vi "main.vi"() -> ()   [LabVIEW 2015, in "lv-example-postgres.lvlib"]
uses:
  lv-example-postgres.lvlib
  private/_controls/timezone.ctl
  <vilib>/addons/database/Connection.llb/Conn ObjectReference.ctl
  <vilib>/addons/database/Connection.llb/Conn Execute.vi
  <vilib>/addons/database/Recordset.llb/Rec Destroy - Connection.vi
  <vilib>/addons/database/Connection.llb/DB Tools Open Connec (String).vi
  <vilib>/addons/database/Command.llb/Cmd Execute.vi
  <vilib>/addons/database/Recordset.llb/Rec Fetch Recordset Data (CR).vi
  <vilib>/addons/database/Recordset.llb/Rec Destroy - Command.vi
  <vilib>/addons/database/Command.llb/Cmd Delete.vi
  <vilib>/addons/database/Recordset.llb/Rec Fetch Recordset Data (R).vi
  <vilib>/addons/database/NI_Database_API.lvlib
panel:
  in  "port":string="5432"
  in  "database":string="postgres"
  in  "display_timezone":i32(ring)=185 items=["Zulu (00:00:00)", "Libya (02:00:00)", "Antarctica/Mawson (05:00:00)", "Antarctica/McMurdo (13:00:00)", "Antarctica/South_Pole (13:00:00)", "Antarctica/Casey (11:00:00)", "Antarctica/Vostok (06:00:00)", "Antarctica/Troll (00:00:00)", "Antarctica/Syowa (03:00:00)", "Antarctica/Macquarie (11:00:00)", "Antarctica/Palmer (-03:00:00)", "Antarctica/DumontDUrville (10:00:00)", "Antarctica/Rothera (-03:00:00)", "Antarctica/Davis (07:00:00)", "NZ-CHAT (13:45:00)", "GMT+0 (00:00:00)", "Cuba (-05:00:00)", "MET (01:00:00)", "Hongkong (08:00:00)", "Poland (01:00:00)", "EST5EDT (-05:00:00)", "EET (02:00:00)", "posix/Zulu (00:00:00)", "posix/Libya (02:00:00)", "posix/Antarctica/Mawson (05:00:00)", "posix/Antarctica/McMurdo (13:00:00)", "posix/Antarctica/South_Pole (13:00:00)", "posix/Antarctica/Casey (11:00:00)", "posix/Antarctica/Vostok (06:00:00)", "posix/Antarctica/Troll (00:00:00)", "posix/Antarctica/Syowa (03:00:00)", "posix/Antarctica/Macquarie (11:00:00)", "posix/Antarctica/Palmer (-03:00:00)", "posix/Antarctica/DumontDUrville (10:00:00)", "posix/Antarctica/Rothera (-03:00:00)", "posix/Antarctica/Davis (07:00:00)", "posix/NZ-CHAT (13:45:00)", "posix/GMT+0 (00:00:00)", "posix/Cuba (-05:00:00)", "posix/MET (01:00:00)", "posix/Hongkong (08:00:00)", "posix/Poland (01:00:00)", "posix/EST5EDT (-05:00:00)", "posix/EET (02:00:00)", "posix/UTC (00:00:00)", "posix/HST (-10:00:00)", "posix/CST6CDT (-06:00:00)", "posix/PRC (08:00:00)", "posix/GB-Eire (00:00:00)", "posix/Australia/Queensland (10:00:00)", "posix/Australia/Currie (11:00:00)", "posix/Australia/Tasmania (11:00:00)", "posix/Australia/South (10:30:00)", "posix/Australia/Victoria (11:00:00)", "posix/Australia/Eucla (08:45:00)", "posix/Australia/Darwin (09:30:00)", "posix/Australia/Hobart (11:00:00)", "posix/Australia/NSW (11:00:00)", "posix/Australia/North (09:30:00)", "posix/Australia/Sydney (11:00:00)", "posix/Australia/Brisbane (10:00:00)", "posix/Australia/Lord_Howe (11:00:00)", "posix/Australia/Perth (08:00:00)", "posix/Australia/Melbourne (11:00:00)", "posix/Australia/LHI (11:00:00)", "posix/Australia/Yancowinna (10:30:00)", "posix/Australia/Lindeman (10:00:00)", "posix/Australia/ACT (11:00:00)", "posix/Australia/Broken_Hill (10:30:00)", "posix/Australia/West (08:00:00)", "posix/Australia/Adelaide (10:30:00)", "posix/Australia/Canberra (11:00:00)", "posix/Europe/Busingen (01:00:00)", "posix/Europe/Gibraltar (01:00:00)", "posix/Europe/San_Marino (01:00:00)", "posix/Europe/Madrid (01:00:00)", "posix/Europe/Helsinki (02:00:00)", "posix/Europe/Brussels (01:00:00)", "posix/Europe/Astrakhan (04:00:00)", "posix/Europe/Belfast (00:00:00)", "posix/Europe/Uzhgorod (02:00:00)", "posix/Europe/Riga (02:00:00)", "posix/Europe/Sarajevo (01:00:00)", "posix/Europe/Vienna (01:00:00)", "posix/Europe/London (00:00:00)", "posix/Europe/Lisbon (00:00:00)", "posix/Europe/Skopje (01:00:00)", "posix/Europe/Monaco (01:00:00)", "posix/Europe/Vaduz (01:00:00)", "posix/Europe/Amsterdam (01:00:00)", "posix/Europe/Kiev (02:00:00)", "posix/Europe/Vilnius (02:00:00)", "posix/Europe/Oslo (01:00:00)", "posix/Europe/Nicosia (02:00:00)", "posix/Europe/Minsk (03:00:00)", "posix/Europe/Budapest (01:00:00)", "posix/Europe/Samara (04:00:00)", "posix/Europe/Kirov (03:00:00)", "posix/Europe/Kaliningrad (02:00:00)", "posix/Europe/Ljubljana (01:00:00)", "posix/Europe/Simferopol (03:00:00)", "posix/Europe/Tiraspol (02:00:00)", "posix/Europe/Stockholm (01:00:00)", "posix/Europe/Isle_of_Man (00:00:00)", "posix/Europe/Guernsey (00:00:00)", "posix/Europe/Belgrade (01:00:00)", "posix/Europe/Zagreb (01:00:00)", "posix/Europe/Rome (01:00:00)", "posix/Europe/Berlin (01:00:00)", "posix/Europe/Ulyanovsk (04:00:00)", "posix/Europe/Mariehamn (02:00:00)", "posix/Europe/Bucharest (02:00:00)", "posix/Europe/Warsaw (01:00:00)", "posix/Europe/Vatican (01:00:00)", "posix/Europe/Dublin (00:00:00)", "posix/Europe/Istanbul (03:00:00)", "posix/Europe/Andorra (01:00:00)", "posix/Europe/Chisinau (02:00:00)", "posix/Europe/Jersey (00:00:00)", "posix/Europe/Zurich (01:00:00)", "posix/Europe/Athens (02:00:00)", "posix/Europe/Paris (01:00:00)", "posix/Europe/Saratov (04:00:00)", "posix/Europe/Prague (01:00:00)", "posix/Europe/Bratislava (01:00:00)", "posix/Europe/Malta (01:00:00)", "posix/Europe/Podgorica (01:00:00)", "posix/Europe/Copenhagen (01:00:00)", "posix/Europe/Moscow (03:00:00)", "posix/Europe/Luxembourg (01:00:00)", "posix/Europe/Zaporozhye (02:00:00)", "posix/Europe/Tirane (01:00:00)", "posix/Europe/Tallinn (02:00:00)", "posix/Europe/Sofia (02:00:00)", "posix/Europe/Volgograd (03:00:00)", "posix/EST (-05:00:00)", "posix/GMT-0 (00:00:00)", "posix/GMT (00:00:00)", "posix/Navajo (-07:00:00)", "posix/Eire (00:00:00)", "posix/Africa/Dar_es_Salaam (03:00:00)", "posix/Africa/Monrovia (00:00:00)", "posix/Africa/Bissau (00:00:00)", "posix/Africa/Juba (02:00:00)", "posix/Africa/Kinshasa (01:00:00)", "posix/Africa/Mogadishu (03:00:00)", "posix/Africa/Ceuta (01:00:00)", "posix/Africa/Asmara (03:00:00)", "posix/Africa/Asmera (03:00:00)", "posix/Africa/Timbuktu (00:00:00)", "posix/Africa/Tripoli (02:00:00)", "posix/Africa/Blantyre (02:00:00)", "posix/Africa/Banjul (00:00:00)", "posix/Africa/Khartoum (02:00:00)", "posix/Africa/Brazzaville (01:00:00)", "posix/Africa/Ouagadougou (00:00:00)", "posix/Africa/Luanda (01:00:00)", "posix/Africa/Conakry (00:00:00)", "posix/Africa/Tunis (01:00:00)", "posix/Africa/Freetown (00:00:00)", "posix/Africa/Maseru (02:00:00)", "posix/Africa/Addis_Ababa (03:00:00)", "posix/Africa/Abidjan (00:00:00)", "posix/Africa/Maputo (02:00:00)", "posix/Africa/Windhoek (02:00:00)", "posix/Africa/Djibouti (03:00:00)", "posix/Africa/Nouakchott (00:00:00)", "posix/Africa/Cairo (02:00:00)", "posix/Africa/Ndjamena (01:00:00)", "posix/Africa/Nairobi (03:00:00)", "posix/Africa/Harare (02:00:00)", "posix/Africa/Bangui (01:00:00)", "posix/Africa/Lome (00:00:00)", "posix/Africa/Lusaka (02:00:00)", "posix/Africa/Lubumbashi (02:00:00)", "posix/Africa/Douala (01:00:00)", "posix/Africa/Bujumbura (02:00:00)", "posix/Africa/Lagos (01:00:00)", "posix/Africa/Dakar (00:00:00)", "posix/Africa/Porto-Novo (01:00:00)", "posix/Africa/Mbabane (02:00:00)", "posix/Africa/Accra (00:00:00)", "posix/Africa/Kigali (02:00:00)", "posix/Africa/Casablanca (01:00:00)", "posix/Africa/Algiers (01:00:00)", "posix/Africa/Malabo (01:00:00)", "posix/Africa/Niamey (01:00:00)", "posix/Africa/Sao_Tome (00:00:00)", "posix/Africa/Libreville (01:00:00)", "posix/Africa/Bamako (00:00:00)", "posix/Africa/El_Aaiun (01:00:00)", "posix/Africa/Gaborone (02:00:00)", "posix/Africa/Johannesburg (02:00:00)", "posix/Africa/Kampala (03:00:00)", "posix/NZ (13:00:00)", "posix/MST (-07:00:00)", "posix/Arctic/Longyearbyen (01:00:00)", "posix/Turkey (03:00:00)", "posix/US/Indiana-Starke (-06:00:00)", "posix/US/Michigan (-05:00:00)", "posix/US/Hawaii (-10:00:00)", "posix/US/East-Indiana (-05:00:00)", "posix/US/Samoa (-11:00:00)", "posix/US/Alaska (-09:00:00)", "posix/US/Aleutian (-10:00:00)", "posix/US/Arizona (-07:00:00)", "posix/US/Mountain (-07:00:00)", "posix/US/Central (-06:00:00)", "posix/US/Eastern (-05:00:00)", "posix/US/Pacific (-08:00:00)", "posix/Canada/Yukon (-07:00:00)", "posix/Canada/Newfoundland (-02:30:00)", "posix/Canada/Atlantic (-04:00:00)", "posix/Canada/Mountain (-07:00:00)", "posix/Canada/Saskatchewan (-06:00:00)", "posix/Canada/Central (-06:00:00)", "posix/Canada/Eastern (-05:00:00)", "posix/Canada/Pacific (-08:00:00)", "posix/Iceland (00:00:00)", "posix/Israel (02:00:00)", "posix/GMT0 (00:00:00)", "posix/Brazil/East (-03:00:00)", "posix/Brazil/Acre (-05:00:00)", "posix/Brazil/DeNoronha (-02:00:00)", "posix/Brazil/West (-04:00:00)", "posix/Japan (09:00:00)", "posix/ROK (09:00:00)", "posix/Atlantic/Faeroe (00:00:00)", "posix/Atlantic/Jan_Mayen (01:00:00)", "posix/Atlantic/Faroe (00:00:00)", "posix/Atlantic/Madeira (00:00:00)", "posix/Atlantic/St_Helena (00:00:00)", "posix/Atlantic/Canary (00:00:00)", "posix/Atlantic/Reykjavik (00:00:00)", "posix/Atlantic/South_Georgia (-02:00:00)", "posix/Atlantic/Stanley (-03:00:00)", "posix/Atlantic/Cape_Verde (-01:00:00)", "posix/Atlantic/Azores (-01:00:00)", "posix/Atlantic/Bermuda (-04:00:00)", "posix/ROC (08:00:00)", "posix/MST7MDT (-07:00:00)", "posix/America/Eirunepe (-05:00:00)", "posix/America/Danmarkshavn (00:00:00)", "posix/America/Santo_Domingo (-04:00:00)", "posix/America/Chicago (-06:00:00)", "posix/America/Jujuy (-03:00:00)", "posix/America/Regina (-06:00:00)", "posix/America/Atikokan (-05:00:00)", "posix/America/Porto_Velho (-04:00:00)", "posix/America/Port_of_Spain (-04:00:00)", "posix/America/Kentucky/Monticello (-05:00:00)", "posix/America/Kentucky/Louisville (-05:00:00)", "posix/America/Anguilla (-04:00:00)", "posix/America/Tegucigalpa (-06:00:00)", "posix/America/Panama (-05:00:00)", "posix/America/Antigua (-04:00:00)", "posix/America/Cancun (-05:00:00)", "posix/America/Araguaina (-03:00:00)", "posix/America/Goose_Bay (-04:00:00)", "posix/America/Coral_Harbour (-05:00:00)", "posix/America/Nipigon (-05:00:00)", "posix/America/New_York (-05:00:00)", "posix/America/Merida (-06:00:00)", "posix/America/Martinique (-04:00:00)", "posix/America/Inuvik (-07:00:00)", "posix/America/Nassau (-05:00:00)", "posix/America/Cuiaba (-04:00:00)", "posix/America/Phoenix (-07:00:00)", "posix/America/Costa_Rica (-06:00:00)", "posix/America/Toronto (-05:00:00)", "posix/America/Guadeloupe (-04:00:00)", "posix/America/Argentina/Jujuy (-03:00:00)", "posix/America/Argentina/Ushuaia (-03:00:00)", "posix/America/Argentina/Rio_Gallegos (-03:00:00)", "posix/America/Argentina/San_Luis (-03:00:00)", "posix/America/Argentina/San_Juan (-03:00:00)", "posix/America/Argentina/Salta (-03:00:00)", "posix/America/Argentina/La_Rioja (-03:00:00)", "posix/America/Argentina/Catamarca (-03:00:00)", "posix/America/Argentina/ComodRivadavia (-03:00:00)", "posix/America/Argentina/Buenos_Aires (-03:00:00)", "posix/America/Argentina/Cordoba (-03:00:00)", "posix/America/Argentina/Tucuman (-03:00:00)", "posix/America/Argentina/Mendoza (-03:00:00)", "posix/America/Mazatlan (-07:00:00)", "posix/America/Paramaribo (-03:00:00)", "posix/America/Nuuk (-03:00:00)", "posix/America/Thule (-04:00:00)", "posix/America/Sao_Paulo (-03:00:00)", "posix/America/Managua (-06:00:00)", "posix/America/Moncton (-04:00:00)", "posix/America/Recife (-03:00:00)", "posix/America/Port-au-Prince (-05:00:00)", "posix/America/Marigot (-04:00:00)", "posix/America/Anchorage (-09:00:00)", "posix/America/Knox_IN (-06:00:00)", "posix/America/Cayenne (-03:00:00)", "posix/America/Mexico_City (-06:00:00)", "posix/America/Santa_Isabel (-08:00:00)", "posix/America/Glace_Bay (-04:00:00)", "posix/America/Chihuahua (-07:00:00)", "posix/America/Montreal (-05:00:00)", "posix/America/Guayaquil (-05:00:00)", "posix/America/Noronha (-02:00:00)", "posix/America/Dawson (-07:00:00)", "posix/America/Belem (-03:00:00)", "posix/America/Guyana (-04:00:00)", "posix/America/Guatemala (-06:00:00)", "posix/America/Boa_Vista (-04:00:00)", "posix/America/St_Vincent (-04:00:00)", "posix/America/Aruba (-04:00:00)", "posix/America/Rosario (-03:00:00)", "posix/America/Matamoros (-06:00:00)", "posix/America/Detroit (-05:00:00)", "posix/America/Lower_Princes (-04:00:00)", "posix/America/St_Barthelemy (-04:00:00)", "posix/America/St_Johns (-02:30:00)", "posix/America/Tortola (-04:00:00)", "posix/America/Rankin_Inlet (-06:00:00)", "posix/America/Blanc-Sablon (-04:00:00)", "posix/America/Punta_Arenas (-03:00:00)", "posix/America/Bahia (-03:00:00)", "posix/America/Godthab (-03:00:00)", "posix/America/Halifax (-04:00:00)", "posix/America/Virgin (-04:00:00)", "posix/America/Grand_Turk (-05:00:00)", "posix/America/Scoresbysund (-01:00:00)", "posix/America/Ojinaga (-07:00:00)", "posix/America/Nome (-09:00:00)", "posix/America/Havana (-05:00:00)", "posix/America/Thunder_Bay (-05:00:00)", "posix/America/Bogota (-05:00:00)", "posix/America/Belize (-06:00:00)", "posix/America/Tijuana (-08:00:00)", "posix/America/Sitka (-09:00:00)", "posix/America/Juneau (-09:00:00)", "posix/America/Shiprock (-07:00:00)", "posix/America/Porto_Acre (-05:00:00)", "posix/America/Monterrey (-06:00:00)", "posix/America/Winnipeg (-06:00:00)", "posix/America/Boise (-07:00:00)", "posix/America/Iqaluit (-05:00:00)", "posix/America/Puerto_Rico (-04:00:00)", "posix/America/Santarem (-03:00:00)", "posix/America/Curacao (-04:00:00)", "posix/America/North_Dakota/Center (-06:00:00)", "posix/America/North_Dakota/New_Salem (-06:00:00)", "posix/America/North_Dakota/Beulah (-06:00:00)", "posix/America/El_Salvador (-06:00:00)", "posix/America/Menominee (-06:00:00)", "posix/America/Montserrat (-04:00:00)", "posix/America/Indianapolis (-05:00:00)", "posix/America/Rainy_River (-06:00:00)", "posix/America/Dominica (-04:00:00)", "posix/America/Fortaleza (-03:00:00)", "posix/America/Cambridge_Bay (-07:00:00)", "posix/America/Fort_Nelson (-07:00:00)", "posix/America/St_Kitts (-04:00:00)", "posix/America/Yellowknife (-07:00:00)", "posix/America/Santiago (-03:00:00)", "posix/America/Maceio (-03:00:00)", "posix/America/Louisville (-05:00:00)", "posix/America/Catamarca (-03:00:00)", "posix/America/Bahia_Banderas (-06:00:00)", "posix/America/Campo_Grande (-04:00:00)", "posix/America/St_Lucia (-04:00:00)", "posix/America/Buenos_Aires (-03:00:00)", "posix/America/Asuncion (-03:00:00)", "posix/America/Hermosillo (-07:00:00)", "posix/America/Cordoba (-03:00:00)", "posix/America/Edmonton (-07:00:00)", "posix/America/Barbados (-04:00:00)", "posix/America/Lima (-05:00:00)", "posix/America/Dawson_Creek (-07:00:00)", "posix/America/Manaus (-04:00:00)", "posix/America/Yakutat (-09:00:00)", "posix/America/Pangnirtung (-05:00:00)", "posix/America/Caracas (-04:00:00)", "posix/America/Rio_Branco (-05:00:00)", "posix/America/Creston (-07:00:00)", "posix/America/Grenada (-04:00:00)", "posix/America/La_Paz (-04:00:00)", "posix/America/Adak (-10:00:00)", "posix/America/Los_Angeles (-08:00:00)", "posix/America/Fort_Wayne (-05:00:00)", "posix/America/Montevideo (-03:00:00)", "posix/America/Whitehorse (-07:00:00)", "posix/America/Jamaica (-05:00:00)", "posix/America/Mendoza (-03:00:00)", "posix/America/Kralendijk (-04:00:00)", "posix/America/St_Thomas (-04:00:00)", "posix/America/Vancouver (-08:00:00)", "posix/America/Ensenada (-08:00:00)", "posix/America/Metlakatla (-09:00:00)", "posix/America/Indiana/Marengo (-05:00:00)", "posix/America/Indiana/Knox (-06:00:00)", "posix/America/Indiana/Tell_City (-06:00:00)", "posix/America/Indiana/Vevay (-05:00:00)", "posix/America/Indiana/Winamac (-05:00:00)", "posix/America/Indiana/Indianapolis (-05:00:00)", "posix/America/Indiana/Vincennes (-05:00:00)", "posix/America/Indiana/Petersburg (-05:00:00)", "posix/America/Cayman (-05:00:00)", "posix/America/Miquelon (-03:00:00)", "posix/America/Swift_Current (-06:00:00)", "posix/America/Resolute (-06:00:00)", "posix/America/Atka (-10:00:00)", "posix/America/Denver (-07:00:00)", "posix/Universal (00:00:00)", "posix/Etc/Zulu (00:00:00)", "posix/Etc/GMT+0 (00:00:00)", "posix/Etc/GMT-12 (12:00:00)", "posix/Etc/GMT-13 (13:00:00)", "posix/Etc/GMT-6 (06:00:00)", "posix/Etc/UTC (00:00:00)", "posix/Etc/GMT-10 (10:00:00)", "posix/Etc/GMT-3 (03:00:00)", "posix/Etc/GMT-0 (00:00:00)", "posix/Etc/GMT-11 (11:00:00)", "posix/Etc/GMT-5 (05:00:00)", "posix/Etc/GMT (00:00:00)", "posix/Etc/GMT-4 (04:00:00)", "posix/Etc/GMT+3 (-03:00:00)", "posix/Etc/GMT+2 (-02:00:00)", "posix/Etc/GMT0 (00:00:00)", "posix/Etc/GMT-1 (01:00:00)", "posix/Etc/Universal (00:00:00)", "posix/Etc/GMT+7 (-07:00:00)", "posix/Etc/GMT-14 (14:00:00)", "posix/Etc/GMT+1 (-01:00:00)", "posix/Etc/Greenwich (00:00:00)", "posix/Etc/GMT+12 (-12:00:00)", "posix/Etc/GMT-2 (02:00:00)", "posix/Etc/GMT+8 (-08:00:00)", "posix/Etc/GMT+9 (-09:00:00)", "posix/Etc/GMT+11 (-11:00:00)", "posix/Etc/UCT (00:00:00)", "posix/Etc/GMT-8 (08:00:00)", "posix/Etc/GMT+6 (-06:00:00)", "posix/Etc/GMT+10 (-10:00:00)", "posix/Etc/GMT+5 (-05:00:00)", "posix/Etc/GMT-9 (09:00:00)", "posix/Etc/GMT+4 (-04:00:00)", "posix/Etc/GMT-7 (07:00:00)", "posix/Indian/Mayotte (03:00:00)", "posix/Indian/Chagos (06:00:00)", "posix/Indian/Christmas (07:00:00)", "posix/Indian/Cocos (06:30:00)", "posix/Indian/Reunion (04:00:00)", "posix/Indian/Mahe (04:00:00)", "posix/Indian/Maldives (05:00:00)", "posix/Indian/Comoro (03:00:00)", "posix/Indian/Kerguelen (05:00:00)", "posix/Indian/Antananarivo (03:00:00)", "posix/Indian/Mauritius (04:00:00)", "posix/Kwajalein (12:00:00)", "posix/Greenwich (00:00:00)", "posix/W-SU (03:00:00)", "posix/UCT (00:00:00)", "posix/Iran (03:30:00)", "posix/Egypt (02:00:00)", "posix/Chile/Continental (-03:00:00)", "posix/Chile/EasterIsland (-05:00:00)", "posix/Asia/Bangkok (07:00:00)", "posix/Asia/Srednekolymsk (11:00:00)", "posix/Asia/Phnom_Penh (07:00:00)", "posix/Asia/Gaza (02:00:00)", "posix/Asia/Qyzylorda (05:00:00)", "posix/Asia/Aden (03:00:00)", "posix/Asia/Chungking (08:00:00)", "posix/Asia/Ulaanbaatar (08:00:00)", "posix/Asia/Kuwait (03:00:00)", "posix/Asia/Dushanbe (05:00:00)", "posix/Asia/Shanghai (08:00:00)", "posix/Asia/Novokuznetsk (07:00:00)", "posix/Asia/Pontianak (07:00:00)", "posix/Asia/Bahrain (03:00:00)", "posix/Asia/Brunei (08:00:00)", "posix/Asia/Dhaka (06:00:00)", "posix/Asia/Bishkek (06:00:00)", "posix/Asia/Barnaul (07:00:00)", "posix/Asia/Ho_Chi_Minh (07:00:00)", "posix/Asia/Macau (08:00:00)", "posix/Asia/Pyongyang (09:00:00)", "posix/Asia/Ashkhabad (05:00:00)", "posix/Asia/Kuala_Lumpur (08:00:00)", "posix/Asia/Yangon (06:30:00)", "posix/Asia/Magadan (11:00:00)", "posix/Asia/Ashgabat (05:00:00)", "posix/Asia/Saigon (07:00:00)", "posix/Asia/Calcutta (05:30:00)", "posix/Asia/Tel_Aviv (02:00:00)", "posix/Asia/Karachi (05:00:00)", "posix/Asia/Atyrau (05:00:00)", "posix/Asia/Samarkand (05:00:00)", "posix/Asia/Taipei (08:00:00)", "posix/Asia/Aqtobe (05:00:00)", "posix/Asia/Riyadh (03:00:00)", "posix/Asia/Almaty (06:00:00)", "posix/Asia/Jakarta (07:00:00)", "posix/Asia/Manila (08:00:00)", "posix/Asia/Nicosia (02:00:00)", "posix/Asia/Novosibirsk (07:00:00)", "posix/Asia/Tokyo (09:00:00)", "posix/Asia/Thimphu (06:00:00)", "posix/Asia/Vientiane (07:00:00)", "posix/Asia/Ulan_Bator (08:00:00)", "posix/Asia/Anadyr (12:00:00)", "posix/Asia/Hovd (07:00:00)", "posix/Asia/Dacca (06:00:00)", "posix/Asia/Beirut (02:00:00)", "posix/Asia/Irkutsk (08:00:00)", "posix/Asia/Yakutsk (09:00:00)", "posix/Asia/Kabul (04:30:00)", "posix/Asia/Tehran (03:30:00)", "posix/Asia/Hong_Kong (08:00:00)", "posix/Asia/Macao (08:00:00)", "posix/Asia/Urumqi (06:00:00)", "posix/Asia/Muscat (04:00:00)", "posix/Asia/Thimbu (06:00:00)", "posix/Asia/Chita (09:00:00)", "posix/Asia/Tomsk (07:00:00)", "posix/Asia/Aqtau (05:00:00)", "posix/Asia/Krasnoyarsk (07:00:00)", "posix/Asia/Kashgar (06:00:00)", "posix/Asia/Kolkata (05:30:00)", "posix/Asia/Kathmandu (05:45:00)", "posix/Asia/Sakhalin (11:00:00)", "posix/Asia/Oral (05:00:00)", "posix/Asia/Tashkent (05:00:00)", "posix/Asia/Istanbul (03:00:00)", "posix/Asia/Dili (09:00:00)", "posix/Asia/Jayapura (09:00:00)", "posix/Asia/Qostanay (06:00:00)", "posix/Asia/Khandyga (09:00:00)", "posix/Asia/Vladivostok (10:00:00)", "posix/Asia/Seoul (09:00:00)", "posix/Asia/Harbin (08:00:00)", "posix/Asia/Amman (02:00:00)", "posix/Asia/Ust-Nera (10:00:00)", "posix/Asia/Qatar (03:00:00)", "posix/Asia/Kuching (08:00:00)", "posix/Asia/Omsk (06:00:00)", "posix/Asia/Baghdad (03:00:00)", "posix/Asia/Choibalsan (08:00:00)", "posix/Asia/Dubai (04:00:00)", "posix/Asia/Chongqing (08:00:00)", "posix/Asia/Makassar (08:00:00)", "posix/Asia/Rangoon (06:30:00)", "posix/Asia/Singapore (08:00:00)", "posix/Asia/Yerevan (04:00:00)", "posix/Asia/Damascus (02:00:00)", "posix/Asia/Tbilisi (04:00:00)", "posix/Asia/Katmandu (05:45:00)", "posix/Asia/Baku (04:00:00)", "posix/Asia/Yekaterinburg (05:00:00)", "posix/Asia/Hebron (02:00:00)", "posix/Asia/Famagusta (02:00:00)", "posix/Asia/Ujung_Pandang (08:00:00)", "posix/Asia/Colombo (05:30:00)", "posix/Asia/Kamchatka (12:00:00)", "posix/Asia/Jerusalem (02:00:00)", "posix/GB (00:00:00)", "posix/Singapore (08:00:00)", "posix/CET (01:00:00)", "posix/Jamaica (-05:00:00)", "posix/PST8PDT (-08:00:00)", "posix/Portugal (00:00:00)", "posix/Pacific/Efate (11:00:00)", "posix/Pacific/Yap (10:00:00)", "posix/Pacific/Wallis (12:00:00)", "posix/Pacific/Saipan (10:00:00)", "posix/Pacific/Tahiti (-10:00:00)", "posix/Pacific/Bougainville (11:00:00)", "posix/Pacific/Pago_Pago (-11:00:00)", "posix/Pacific/Niue (-11:00:00)", "posix/Pacific/Honolulu (-10:00:00)", "posix/Pacific/Samoa (-11:00:00)", "posix/Pacific/Enderbury (13:00:00)", "posix/Pacific/Pitcairn (-08:00:00)", "posix/Pacific/Johnston (-10:00:00)", "posix/Pacific/Funafuti (12:00:00)", "posix/Pacific/Norfolk (12:00:00)", "posix/Pacific/Tongatapu (13:00:00)", "posix/Pacific/Apia (13:00:00)", "posix/Pacific/Truk (10:00:00)", "posix/Pacific/Guam (10:00:00)", "posix/Pacific/Nauru (12:00:00)", "posix/Pacific/Palau (09:00:00)", "posix/Pacific/Chatham (13:45:00)", "posix/Pacific/Rarotonga (-10:00:00)", "posix/Pacific/Majuro (12:00:00)", "posix/Pacific/Wake (12:00:00)", "posix/Pacific/Gambier (-09:00:00)", "posix/Pacific/Auckland (13:00:00)", "posix/Pacific/Pohnpei (11:00:00)", "posix/Pacific/Midway (-11:00:00)", "posix/Pacific/Fiji (13:00:00)", "posix/Pacific/Marquesas (-08:30:00)", "posix/Pacific/Ponape (11:00:00)", "posix/Pacific/Port_Moresby (10:00:00)", "posix/Pacific/Noumea (11:00:00)", "posix/Pacific/Kwajalein (12:00:00)", "posix/Pacific/Tarawa (12:00:00)", "posix/Pacific/Easter (-05:00:00)", "posix/Pacific/Chuuk (10:00:00)", "posix/Pacific/Kiritimati (14:00:00)", "posix/Pacific/Guadalcanal (11:00:00)", "posix/Pacific/Galapagos (-06:00:00)", "posix/Pacific/Fakaofo (13:00:00)", "posix/Pacific/Kosrae (11:00:00)", "posix/Factory (00:00:00)", "posix/WET (00:00:00)", "posix/Mexico/BajaSur (-07:00:00)", "posix/Mexico/BajaNorte (-08:00:00)", "posix/Mexico/General (-06:00:00)", "UTC (00:00:00)", "HST (-10:00:00)", "CST6CDT (-06:00:00)", "PRC (08:00:00)", "GB-Eire (00:00:00)", "Australia/Queensland (10:00:00)", "Australia/Currie (11:00:00)", "Australia/Tasmania (11:00:00)", "Australia/South (10:30:00)", "Australia/Victoria (11:00:00)", "Australia/Eucla (08:45:00)", "Australia/Darwin (09:30:00)", "Australia/Hobart (11:00:00)", "Australia/NSW (11:00:00)", "Australia/North (09:30:00)", "Australia/Sydney (11:00:00)", "Australia/Brisbane (10:00:00)", "Australia/Lord_Howe (11:00:00)", "Australia/Perth (08:00:00)", "Australia/Melbourne (11:00:00)", "Australia/LHI (11:00:00)", "Australia/Yancowinna (10:30:00)", "Australia/Lindeman (10:00:00)", "Australia/ACT (11:00:00)", "Australia/Broken_Hill (10:30:00)", "Australia/West (08:00:00)", "Australia/Adelaide (10:30:00)", "Australia/Canberra (11:00:00)", "Europe/Busingen (01:00:00)", "Europe/Gibraltar (01:00:00)", "Europe/San_Marino (01:00:00)", "Europe/Madrid (01:00:00)", "Europe/Helsinki (02:00:00)", "Europe/Brussels (01:00:00)", "Europe/Astrakhan (04:00:00)", "Europe/Belfast (00:00:00)", "Europe/Uzhgorod (02:00:00)", "Europe/Riga (02:00:00)", "Europe/Sarajevo (01:00:00)", "Europe/Vienna (01:00:00)", "Europe/London (00:00:00)", "Europe/Lisbon (00:00:00)", "Europe/Skopje (01:00:00)", "Europe/Monaco (01:00:00)", "Europe/Vaduz (01:00:00)", "Europe/Amsterdam (01:00:00)", "Europe/Kiev (02:00:00)", "Europe/Vilnius (02:00:00)", "Europe/Oslo (01:00:00)", "Europe/Nicosia (02:00:00)", "Europe/Minsk (03:00:00)", "Europe/Budapest (01:00:00)", "Europe/Samara (04:00:00)", "Europe/Kirov (03:00:00)", "Europe/Kaliningrad (02:00:00)", "Europe/Ljubljana (01:00:00)", "Europe/Simferopol (03:00:00)", "Europe/Tiraspol (02:00:00)", "Europe/Stockholm (01:00:00)", "Europe/Isle_of_Man (00:00:00)", "Europe/Guernsey (00:00:00)", "Europe/Belgrade (01:00:00)", "Europe/Zagreb (01:00:00)", "Europe/Rome (01:00:00)", "Europe/Berlin (01:00:00)", "Europe/Ulyanovsk (04:00:00)", "Europe/Mariehamn (02:00:00)", "Europe/Bucharest (02:00:00)", "Europe/Warsaw (01:00:00)", "Europe/Vatican (01:00:00)", "Europe/Dublin (00:00:00)", "Europe/Istanbul (03:00:00)", "Europe/Andorra (01:00:00)", "Europe/Chisinau (02:00:00)", "Europe/Jersey (00:00:00)", "Europe/Zurich (01:00:00)", "Europe/Athens (02:00:00)", "Europe/Paris (01:00:00)", "Europe/Saratov (04:00:00)", "Europe/Prague (01:00:00)", "Europe/Bratislava (01:00:00)", "Europe/Malta (01:00:00)", "Europe/Podgorica (01:00:00)", "Europe/Copenhagen (01:00:00)", "Europe/Moscow (03:00:00)", "Europe/Luxembourg (01:00:00)", "Europe/Zaporozhye (02:00:00)", "Europe/Tirane (01:00:00)", "Europe/Tallinn (02:00:00)", "Europe/Sofia (02:00:00)", "Europe/Volgograd (03:00:00)", "EST (-05:00:00)", "GMT-0 (00:00:00)", "GMT (00:00:00)", "Navajo (-07:00:00)", "Eire (00:00:00)", "Africa/Dar_es_Salaam (03:00:00)", "Africa/Monrovia (00:00:00)", "Africa/Bissau (00:00:00)", "Africa/Juba (02:00:00)", "Africa/Kinshasa (01:00:00)", "Africa/Mogadishu (03:00:00)", "Africa/Ceuta (01:00:00)", "Africa/Asmara (03:00:00)", "Africa/Asmera (03:00:00)", "Africa/Timbuktu (00:00:00)", "Africa/Tripoli (02:00:00)", "Africa/Blantyre (02:00:00)", "Africa/Banjul (00:00:00)", "Africa/Khartoum (02:00:00)", "Africa/Brazzaville (01:00:00)", "Africa/Ouagadougou (00:00:00)", "Africa/Luanda (01:00:00)", "Africa/Conakry (00:00:00)", "Africa/Tunis (01:00:00)", "Africa/Freetown (00:00:00)", "Africa/Maseru (02:00:00)", "Africa/Addis_Ababa (03:00:00)", "Africa/Abidjan (00:00:00)", "Africa/Maputo (02:00:00)", "Africa/Windhoek (02:00:00)", "Africa/Djibouti (03:00:00)", "Africa/Nouakchott (00:00:00)", "Africa/Cairo (02:00:00)", "Africa/Ndjamena (01:00:00)", "Africa/Nairobi (03:00:00)", "Africa/Harare (02:00:00)", "Africa/Bangui (01:00:00)", "Africa/Lome (00:00:00)", "Africa/Lusaka (02:00:00)", "Africa/Lubumbashi (02:00:00)", "Africa/Douala (01:00:00)", "Africa/Bujumbura (02:00:00)", "Africa/Lagos (01:00:00)", "Africa/Dakar (00:00:00)", "Africa/Porto-Novo (01:00:00)", "Africa/Mbabane (02:00:00)", "Africa/Accra (00:00:00)", "Africa/Kigali (02:00:00)", "Africa/Casablanca (01:00:00)", "Africa/Algiers (01:00:00)", "Africa/Malabo (01:00:00)", "Africa/Niamey (01:00:00)", "Africa/Sao_Tome (00:00:00)", "Africa/Libreville (01:00:00)", "Africa/Bamako (00:00:00)", "Africa/El_Aaiun (01:00:00)", "Africa/Gaborone (02:00:00)", "Africa/Johannesburg (02:00:00)", "Africa/Kampala (03:00:00)", "NZ (13:00:00)", "MST (-07:00:00)", "Arctic/Longyearbyen (01:00:00)", "Turkey (03:00:00)", "US/Indiana-Starke (-06:00:00)", "US/Michigan (-05:00:00)", "US/Hawaii (-10:00:00)", "US/East-Indiana (-05:00:00)", "US/Samoa (-11:00:00)", "US/Alaska (-09:00:00)", "US/Aleutian (-10:00:00)", "US/Arizona (-07:00:00)", "US/Mountain (-07:00:00)", "US/Central (-06:00:00)", "US/Eastern (-05:00:00)", "US/Pacific (-08:00:00)", "Canada/Yukon (-07:00:00)", "Canada/Newfoundland (-02:30:00)", "Canada/Atlantic (-04:00:00)", "Canada/Mountain (-07:00:00)", "Canada/Saskatchewan (-06:00:00)", "Canada/Central (-06:00:00)", "Canada/Eastern (-05:00:00)", "Canada/Pacific (-08:00:00)", "Iceland (00:00:00)", "Israel (02:00:00)", "GMT0 (00:00:00)", "Brazil/East (-03:00:00)", "Brazil/Acre (-05:00:00)", "Brazil/DeNoronha (-02:00:00)", "Brazil/West (-04:00:00)", "Japan (09:00:00)", "ROK (09:00:00)", "Atlantic/Faeroe (00:00:00)", "Atlantic/Jan_Mayen (01:00:00)", "Atlantic/Faroe (00:00:00)", "Atlantic/Madeira (00:00:00)", "Atlantic/St_Helena (00:00:00)", "Atlantic/Canary (00:00:00)", "Atlantic/Reykjavik (00:00:00)", "Atlantic/South_Georgia (-02:00:00)", "Atlantic/Stanley (-03:00:00)", "Atlantic/Cape_Verde (-01:00:00)", "Atlantic/Azores (-01:00:00)", "Atlantic/Bermuda (-04:00:00)", "ROC (08:00:00)", "MST7MDT (-07:00:00)", "America/Eirunepe (-05:00:00)", "America/Danmarkshavn (00:00:00)", "America/Santo_Domingo (-04:00:00)", "America/Chicago (-06:00:00)", "America/Jujuy (-03:00:00)", "America/Regina (-06:00:00)", "America/Atikokan (-05:00:00)", "America/Porto_Velho (-04:00:00)", "America/Port_of_Spain (-04:00:00)", "America/Kentucky/Monticello (-05:00:00)", "America/Kentucky/Louisville (-05:00:00)", "America/Anguilla (-04:00:00)", "America/Tegucigalpa (-06:00:00)", "America/Panama (-05:00:00)", "America/Antigua (-04:00:00)", "America/Cancun (-05:00:00)", "America/Araguaina (-03:00:00)", "America/Goose_Bay (-04:00:00)", "America/Coral_Harbour (-05:00:00)", "America/Nipigon (-05:00:00)", "America/New_York (-05:00:00)", "America/Merida (-06:00:00)", "America/Martinique (-04:00:00)", "America/Inuvik (-07:00:00)", "America/Nassau (-05:00:00)", "America/Cuiaba (-04:00:00)", "America/Phoenix (-07:00:00)", "America/Costa_Rica (-06:00:00)", "America/Toronto (-05:00:00)", "America/Guadeloupe (-04:00:00)", "America/Argentina/Jujuy (-03:00:00)", "America/Argentina/Ushuaia (-03:00:00)", "America/Argentina/Rio_Gallegos (-03:00:00)", "America/Argentina/San_Luis (-03:00:00)", "America/Argentina/San_Juan (-03:00:00)", "America/Argentina/Salta (-03:00:00)", "America/Argentina/La_Rioja (-03:00:00)", "America/Argentina/Catamarca (-03:00:00)", "America/Argentina/ComodRivadavia (-03:00:00)", "America/Argentina/Buenos_Aires (-03:00:00)", "America/Argentina/Cordoba (-03:00:00)", "America/Argentina/Tucuman (-03:00:00)", "America/Argentina/Mendoza (-03:00:00)", "America/Mazatlan (-07:00:00)", "America/Paramaribo (-03:00:00)", "America/Nuuk (-03:00:00)", "America/Thule (-04:00:00)", "America/Sao_Paulo (-03:00:00)", "America/Managua (-06:00:00)", "America/Moncton (-04:00:00)", "America/Recife (-03:00:00)", "America/Port-au-Prince (-05:00:00)", "America/Marigot (-04:00:00)", "America/Anchorage (-09:00:00)", "America/Knox_IN (-06:00:00)", "America/Cayenne (-03:00:00)", "America/Mexico_City (-06:00:00)", "America/Santa_Isabel (-08:00:00)", "America/Glace_Bay (-04:00:00)", "America/Chihuahua (-07:00:00)", "America/Montreal (-05:00:00)", "America/Guayaquil (-05:00:00)", "America/Noronha (-02:00:00)", "America/Dawson (-07:00:00)", "America/Belem (-03:00:00)", "America/Guyana (-04:00:00)", "America/Guatemala (-06:00:00)", "America/Boa_Vista (-04:00:00)", "America/St_Vincent (-04:00:00)", "America/Aruba (-04:00:00)", "America/Rosario (-03:00:00)", "America/Matamoros (-06:00:00)", "America/Detroit (-05:00:00)", "America/Lower_Princes (-04:00:00)", "America/St_Barthelemy (-04:00:00)", "America/St_Johns (-02:30:00)", "America/Tortola (-04:00:00)", "America/Rankin_Inlet (-06:00:00)", "America/Blanc-Sablon (-04:00:00)", "America/Punta_Arenas (-03:00:00)", "America/Bahia (-03:00:00)", "America/Godthab (-03:00:00)", "America/Halifax (-04:00:00)", "America/Virgin (-04:00:00)", "America/Grand_Turk (-05:00:00)", "America/Scoresbysund (-01:00:00)", "America/Ojinaga (-07:00:00)", "America/Nome (-09:00:00)", "America/Havana (-05:00:00)", "America/Thunder_Bay (-05:00:00)", "America/Bogota (-05:00:00)", "America/Belize (-06:00:00)", "America/Tijuana (-08:00:00)", "America/Sitka (-09:00:00)", "America/Juneau (-09:00:00)", "America/Shiprock (-07:00:00)", "America/Porto_Acre (-05:00:00)", "America/Monterrey (-06:00:00)", "America/Winnipeg (-06:00:00)", "America/Boise (-07:00:00)", "America/Iqaluit (-05:00:00)", "America/Puerto_Rico (-04:00:00)", "America/Santarem (-03:00:00)", "America/Curacao (-04:00:00)", "America/North_Dakota/Center (-06:00:00)", "America/North_Dakota/New_Salem (-06:00:00)", "America/North_Dakota/Beulah (-06:00:00)", "America/El_Salvador (-06:00:00)", "America/Menominee (-06:00:00)", "America/Montserrat (-04:00:00)", "America/Indianapolis (-05:00:00)", "America/Rainy_River (-06:00:00)", "America/Dominica (-04:00:00)", "America/Fortaleza (-03:00:00)", "America/Cambridge_Bay (-07:00:00)", "America/Fort_Nelson (-07:00:00)", "America/St_Kitts (-04:00:00)", "America/Yellowknife (-07:00:00)", "America/Santiago (-03:00:00)", "America/Maceio (-03:00:00)", "America/Louisville (-05:00:00)", "America/Catamarca (-03:00:00)", "America/Bahia_Banderas (-06:00:00)", "America/Campo_Grande (-04:00:00)", "America/St_Lucia (-04:00:00)", "America/Buenos_Aires (-03:00:00)", "America/Asuncion (-03:00:00)", "America/Hermosillo (-07:00:00)", "America/Cordoba (-03:00:00)", "America/Edmonton (-07:00:00)", "America/Barbados (-04:00:00)", "America/Lima (-05:00:00)", "America/Dawson_Creek (-07:00:00)", "America/Manaus (-04:00:00)", "America/Yakutat (-09:00:00)", "America/Pangnirtung (-05:00:00)", "America/Caracas (-04:00:00)", "America/Rio_Branco (-05:00:00)", "America/Creston (-07:00:00)", "America/Grenada (-04:00:00)", "America/La_Paz (-04:00:00)", "America/Adak (-10:00:00)", "America/Los_Angeles (-08:00:00)", "America/Fort_Wayne (-05:00:00)", "America/Montevideo (-03:00:00)", "America/Whitehorse (-07:00:00)", "America/Jamaica (-05:00:00)", "America/Mendoza (-03:00:00)", "America/Kralendijk (-04:00:00)", "America/St_Thomas (-04:00:00)", "America/Vancouver (-08:00:00)", "America/Ensenada (-08:00:00)", "America/Metlakatla (-09:00:00)", "America/Indiana/Marengo (-05:00:00)", "America/Indiana/Knox (-06:00:00)", "America/Indiana/Tell_City (-06:00:00)", "America/Indiana/Vevay (-05:00:00)", "America/Indiana/Winamac (-05:00:00)", "America/Indiana/Indianapolis (-05:00:00)", "America/Indiana/Vincennes (-05:00:00)", "America/Indiana/Petersburg (-05:00:00)", "America/Cayman (-05:00:00)", "America/Miquelon (-03:00:00)", "America/Swift_Current (-06:00:00)", "America/Resolute (-06:00:00)", "America/Atka (-10:00:00)", "America/Denver (-07:00:00)", "Universal (00:00:00)", "Etc/Zulu (00:00:00)", "Etc/GMT+0 (00:00:00)", "Etc/GMT-12 (12:00:00)", "Etc/GMT-13 (13:00:00)", "Etc/GMT-6 (06:00:00)", "Etc/UTC (00:00:00)", "Etc/GMT-10 (10:00:00)", "Etc/GMT-3 (03:00:00)", "Etc/GMT-0 (00:00:00)", "Etc/GMT-11 (11:00:00)", "Etc/GMT-5 (05:00:00)", "Etc/GMT (00:00:00)", "Etc/GMT-4 (04:00:00)", "Etc/GMT+3 (-03:00:00)", "Etc/GMT+2 (-02:00:00)", "Etc/GMT0 (00:00:00)", "Etc/GMT-1 (01:00:00)", "Etc/Universal (00:00:00)", "Etc/GMT+7 (-07:00:00)", "Etc/GMT-14 (14:00:00)", "Etc/GMT+1 (-01:00:00)", "Etc/Greenwich (00:00:00)", "Etc/GMT+12 (-12:00:00)", "Etc/GMT-2 (02:00:00)", "Etc/GMT+8 (-08:00:00)", "Etc/GMT+9 (-09:00:00)", "Etc/GMT+11 (-11:00:00)", "Etc/UCT (00:00:00)", "Etc/GMT-8 (08:00:00)", "Etc/GMT+6 (-06:00:00)", "Etc/GMT+10 (-10:00:00)", "Etc/GMT+5 (-05:00:00)", "Etc/GMT-9 (09:00:00)", "Etc/GMT+4 (-04:00:00)", "Etc/GMT-7 (07:00:00)", "Indian/Mayotte (03:00:00)", "Indian/Chagos (06:00:00)", "Indian/Christmas (07:00:00)", "Indian/Cocos (06:30:00)", "Indian/Reunion (04:00:00)", "Indian/Mahe (04:00:00)", "Indian/Maldives (05:00:00)", "Indian/Comoro (03:00:00)", "Indian/Kerguelen (05:00:00)", "Indian/Antananarivo (03:00:00)", "Indian/Mauritius (04:00:00)", "Kwajalein (12:00:00)", "Greenwich (00:00:00)", "W-SU (03:00:00)", "UCT (00:00:00)", "Iran (03:30:00)", "Egypt (02:00:00)", "Chile/Continental (-03:00:00)", "Chile/EasterIsland (-05:00:00)", "Asia/Bangkok (07:00:00)", "Asia/Srednekolymsk (11:00:00)", "Asia/Phnom_Penh (07:00:00)", "Asia/Gaza (02:00:00)", "Asia/Qyzylorda (05:00:00)", "Asia/Aden (03:00:00)", "Asia/Chungking (08:00:00)", "Asia/Ulaanbaatar (08:00:00)", "Asia/Kuwait (03:00:00)", "Asia/Dushanbe (05:00:00)", "Asia/Shanghai (08:00:00)", "Asia/Novokuznetsk (07:00:00)", "Asia/Pontianak (07:00:00)", "Asia/Bahrain (03:00:00)", "Asia/Brunei (08:00:00)", "Asia/Dhaka (06:00:00)", "Asia/Bishkek (06:00:00)", "Asia/Barnaul (07:00:00)", "Asia/Ho_Chi_Minh (07:00:00)", "Asia/Macau (08:00:00)", "Asia/Pyongyang (09:00:00)", "Asia/Ashkhabad (05:00:00)", "Asia/Kuala_Lumpur (08:00:00)", "Asia/Yangon (06:30:00)", "Asia/Magadan (11:00:00)", "Asia/Ashgabat (05:00:00)", "Asia/Saigon (07:00:00)", "Asia/Calcutta (05:30:00)", "Asia/Tel_Aviv (02:00:00)", "Asia/Karachi (05:00:00)", "Asia/Atyrau (05:00:00)", "Asia/Samarkand (05:00:00)", "Asia/Taipei (08:00:00)", "Asia/Aqtobe (05:00:00)", "Asia/Riyadh (03:00:00)", "Asia/Almaty (06:00:00)", "Asia/Jakarta (07:00:00)", "Asia/Manila (08:00:00)", "Asia/Nicosia (02:00:00)", "Asia/Novosibirsk (07:00:00)", "Asia/Tokyo (09:00:00)", "Asia/Thimphu (06:00:00)", "Asia/Vientiane (07:00:00)", "Asia/Ulan_Bator (08:00:00)", "Asia/Anadyr (12:00:00)", "Asia/Hovd (07:00:00)", "Asia/Dacca (06:00:00)", "Asia/Beirut (02:00:00)", "Asia/Irkutsk (08:00:00)", "Asia/Yakutsk (09:00:00)", "Asia/Kabul (04:30:00)", "Asia/Tehran (03:30:00)", "Asia/Hong_Kong (08:00:00)", "Asia/Macao (08:00:00)", "Asia/Urumqi (06:00:00)", "Asia/Muscat (04:00:00)", "Asia/Thimbu (06:00:00)", "Asia/Chita (09:00:00)", "Asia/Tomsk (07:00:00)", "Asia/Aqtau (05:00:00)", "Asia/Krasnoyarsk (07:00:00)", "Asia/Kashgar (06:00:00)", "Asia/Kolkata (05:30:00)", "Asia/Kathmandu (05:45:00)", "Asia/Sakhalin (11:00:00)", "Asia/Oral (05:00:00)", "Asia/Tashkent (05:00:00)", "Asia/Istanbul (03:00:00)", "Asia/Dili (09:00:00)", "Asia/Jayapura (09:00:00)", "Asia/Qostanay (06:00:00)", "Asia/Khandyga (09:00:00)", "Asia/Vladivostok (10:00:00)", "Asia/Seoul (09:00:00)", "Asia/Harbin (08:00:00)", "Asia/Amman (02:00:00)", "Asia/Ust-Nera (10:00:00)", "Asia/Qatar (03:00:00)", "Asia/Kuching (08:00:00)", "Asia/Omsk (06:00:00)", "Asia/Baghdad (03:00:00)", "Asia/Choibalsan (08:00:00)", "Asia/Dubai (04:00:00)", "Asia/Chongqing (08:00:00)", "Asia/Makassar (08:00:00)", "Asia/Rangoon (06:30:00)", "Asia/Singapore (08:00:00)", "Asia/Yerevan (04:00:00)", "Asia/Damascus (02:00:00)", "Asia/Tbilisi (04:00:00)", "Asia/Katmandu (05:45:00)", "Asia/Baku (04:00:00)", "Asia/Yekaterinburg (05:00:00)", "Asia/Hebron (02:00:00)", "Asia/Famagusta (02:00:00)", "Asia/Ujung_Pandang (08:00:00)", "Asia/Colombo (05:30:00)", "Asia/Kamchatka (12:00:00)", "Asia/Jerusalem (02:00:00)", "GB (00:00:00)", "Singapore (08:00:00)", "CET (01:00:00)", "posixrules (-05:00:00)", "Jamaica (-05:00:00)", "PST8PDT (-08:00:00)", "Portugal (00:00:00)", "Pacific/Efate (11:00:00)", "Pacific/Yap (10:00:00)", "Pacific/Wallis (12:00:00)", "Pacific/Saipan (10:00:00)", "Pacific/Tahiti (-10:00:00)", "Pacific/Bougainville (11:00:00)", "Pacific/Pago_Pago (-11:00:00)", "Pacific/Niue (-11:00:00)", "Pacific/Honolulu (-10:00:00)", "Pacific/Samoa (-11:00:00)", "Pacific/Enderbury (13:00:00)", "Pacific/Pitcairn (-08:00:00)", "Pacific/Johnston (-10:00:00)", "Pacific/Funafuti (12:00:00)", "Pacific/Norfolk (12:00:00)", "Pacific/Tongatapu (13:00:00)", "Pacific/Apia (13:00:00)", "Pacific/Truk (10:00:00)", "Pacific/Guam (10:00:00)", "Pacific/Nauru (12:00:00)", "Pacific/Palau (09:00:00)", "Pacific/Chatham (13:45:00)", "Pacific/Rarotonga (-10:00:00)", "Pacific/Majuro (12:00:00)", "Pacific/Wake (12:00:00)", "Pacific/Gambier (-09:00:00)", "Pacific/Auckland (13:00:00)", "Pacific/Pohnpei (11:00:00)", "Pacific/Midway (-11:00:00)", "Pacific/Fiji (13:00:00)", "Pacific/Marquesas (-08:30:00)", "Pacific/Ponape (11:00:00)", "Pacific/Port_Moresby (10:00:00)", "Pacific/Noumea (11:00:00)", "Pacific/Kwajalein (12:00:00)", "Pacific/Tarawa (12:00:00)", "Pacific/Easter (-05:00:00)", "Pacific/Chuuk (10:00:00)", "Pacific/Kiritimati (14:00:00)", "Pacific/Guadalcanal (11:00:00)", "Pacific/Galapagos (-06:00:00)", "Pacific/Fakaofo (13:00:00)", "Pacific/Kosrae (11:00:00)", "Factory (00:00:00)", "WET (00:00:00)", "Mexico/BajaSur (-07:00:00)", "Mexico/BajaNorte (-08:00:00)", "Mexico/General (-06:00:00)", "localtime (00:00:00)"]
  in  "disconnect":bool
  in  "username":string="postgres"
  in  "password":string="postgres"
  in  "server":string="localhost:5432"
  in  "connect":bool
  in  "driver":string="PostgreSQL ANSI"
  out "connected?":bool
  in  "tab_control":T1(tab)
  out "time_display":timestamp format="%^<%H:%M:%S%4u\n%m/%d/%y>T"
  out "time_local":timestamp format="%<%H:%M:%S%4u\n%m/%d/%y>T"
  out "time_utc":timestamp format="%^<%H:%M:%S%4u\n%m/%d/%y>T"
  in  "select_time_now":bool
  in  "clear_table":bool
  out "create_table_sql":string="-- DROP TABLE timeseries\nCREATE TABLE timeseries (\n\ttime timestamp,\n\tvalue double precision,\n    PRIMARY KEY (time)\n);"
  in  "create_table":bool
  out "timezone_names []":string[](array[string])
  out "timezone_offset":dbl format="%<%H:%M:%S>t"
  out "server_timezone":string
  out "timezones":T2[](array[typedef]) {"utc_offset" format="%<%H:%M:%S>t"}
  in  "get_timezones":bool
  out "time_to_insert":dbl format="%<%H:%M:%S%4u>t"
  in  "rate_s":dbl=1.0 format="%<%S%4u>t"
  in  "n_data_points":i32=60
  in  "insert_multiple_data":bool
  out "data_inserted":cluster{"time":dbl, "value":dbl}[](array[cluster]) {"value" format="%#_10f"; "time" format="%^<%H:%M:%S%4u %m/%d/%y>T"}
  in  "clear_inserted_data":bool
  in  "insert_single_data":bool
  in  "reset_ranges":bool
  in  "range_finish":dbl format="%<%H:%M:%S%4u %m/%d/%y>T"
  in  "range_start":dbl format="%<%H:%M:%S%4u %m/%d/%y>T"
  in  "read_data":bool
  out "time_to_read":dbl format="%<%H:%M:%S%4u>t"
  in  "time_selection":T3(ring)=enum."Local"
  out "tab_control_data_read":enum32{"utc", "local"}(tab)
  out "data_read_utc":cluster{"time":dbl, "value":dbl}[](array[cluster]) {"value" format="%#_10f"; "time" format="%^<%H:%M:%S%4u %m/%d/%y>T"}
  out "data_read_local":cluster{"time":dbl, "value":dbl}[](array[cluster]) {"value" format="%#_10f"; "time" format="%<%H:%M:%S%4u %m/%d/%y>T"}
  in  "stop":bool
  out "error":errorcluster
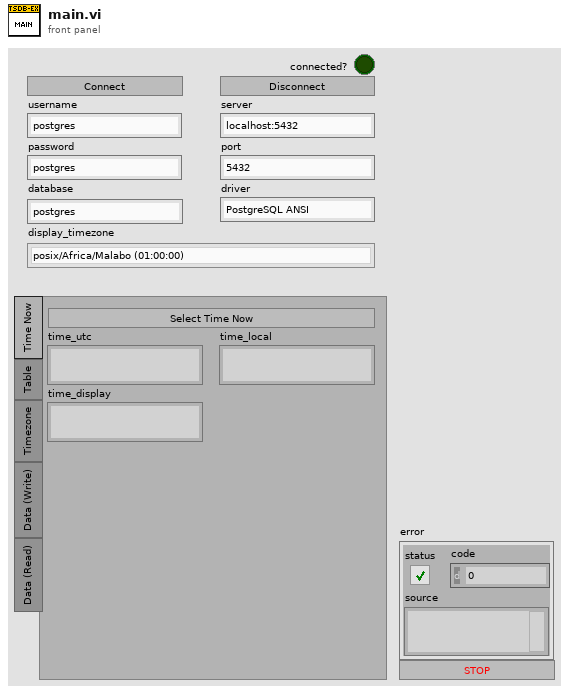
[diagram p1: front panel]
types:
  T1 = enum32{"Time Now", "Table", "Timezone", "Data (Write)", "Data (Read)"}
  T2 = typedef "lv-example-postgres.lvlib/timezone.ctl" = cluster{"name":string, "abbreviation":string, "utc_offset":dbl, "is_dst":bool}
  T3 = enum16{"<time_selection>", "Local", "UTC (Universal Coordinated Time)", "Display Timezone", "<null>"}
  T4 = typedef "NI_Database_API.lvlib/Conn ObjectReference.ctl" = refnum<k1>
  T5 = typedef "NI_Database_API.lvlib/Rec ObjectReference.ctl" = refnum<k1>
  T6 = typedef "NI_Database_API.lvlib/DB Tools Parameter Info.ctl" = cluster{"parameter name":string, "type":T7, "direction":T8, "value":variant}
  T7 = typedef "NI_Database_API.lvlib/DB Tools DataTypes.ctl" = enum16{"String", "Long (I32)", "Single (SGL)", "Double (DBL)", "Date/Time", "Binary"}
  T8 = typedef "NI_Database_API.lvlib/DB Tools Parameter Dir.ctl" = enum32{"Input", "Output", "Input/Output", "Return Value"}
  T9 = typedef "NI_Database_API.lvlib/Cmd ObjectReference.ctl" = refnum<k1>
  T10 = typedef "NI_Database_API.lvlib/Cmd-Rec Object Reference.ctl" = refnum<k1>
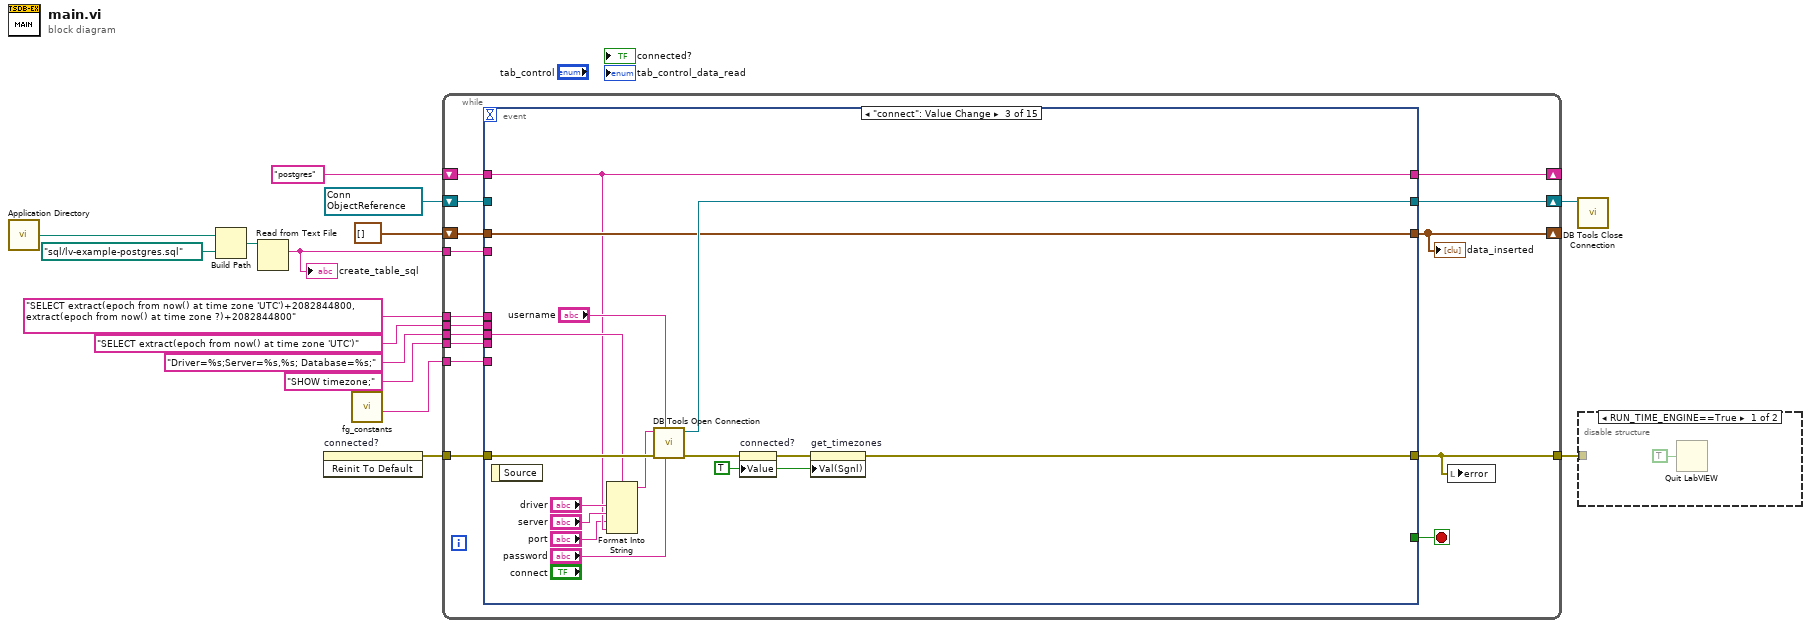
[diagram p0: block diagram]
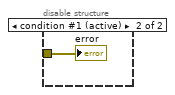
[diagram p2: hidden frame]
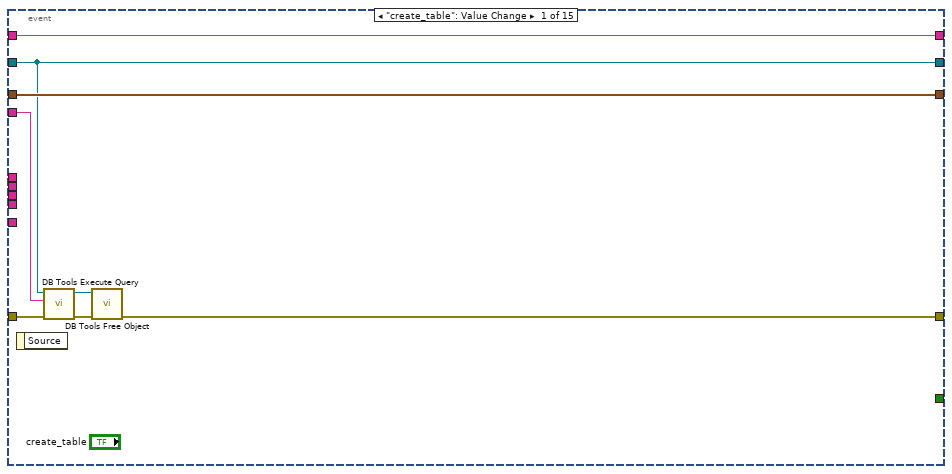
[diagram p3: hidden frame]
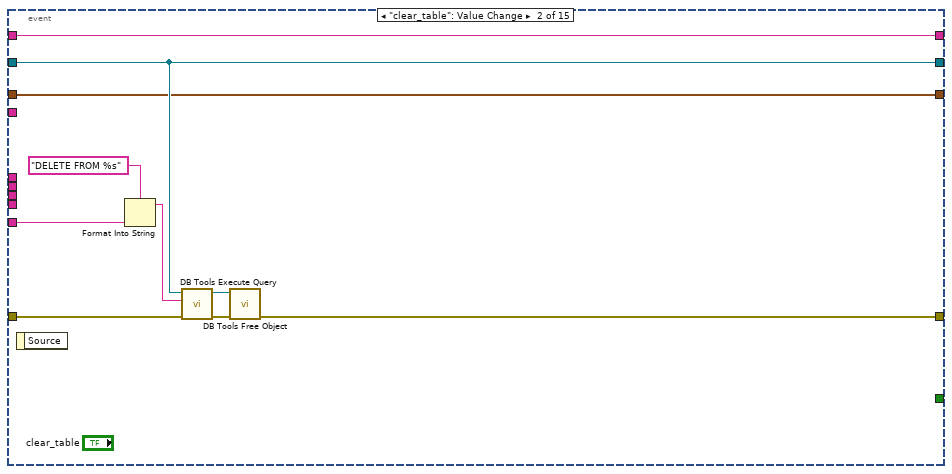
[diagram p4: hidden frame]
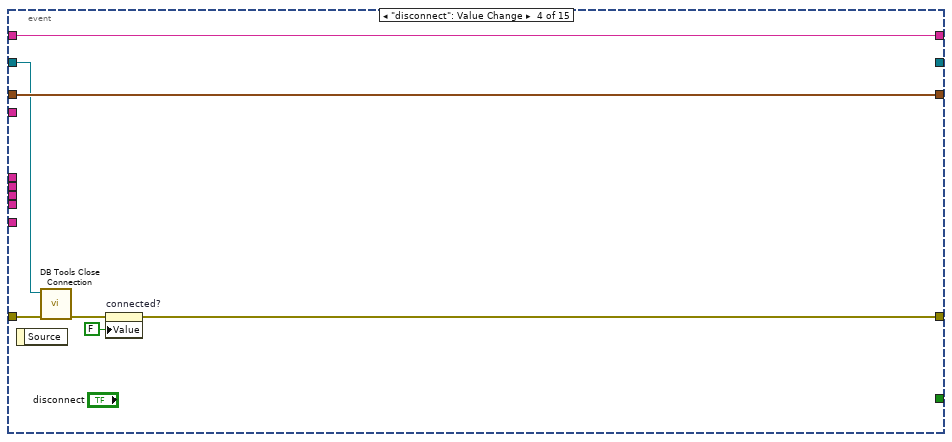
[diagram p5: hidden frame]
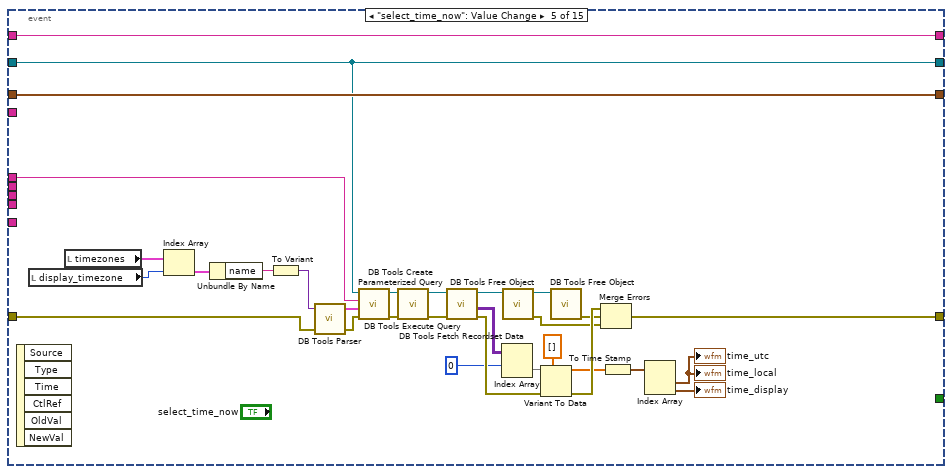
[diagram p6: hidden frame]
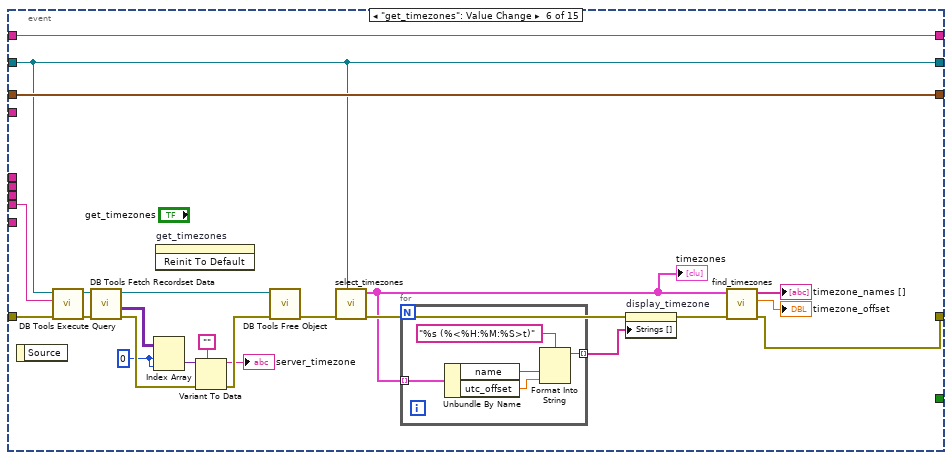
[diagram p7: hidden frame]
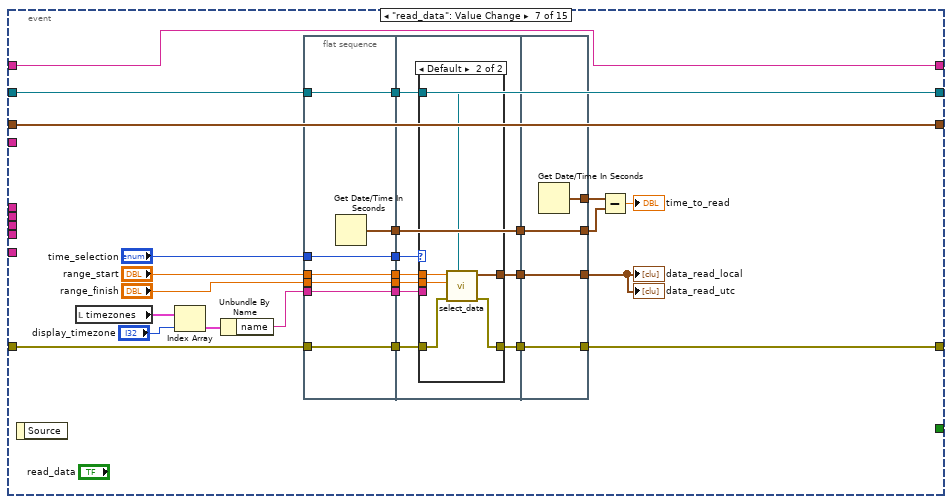
[diagram p8: hidden frame]
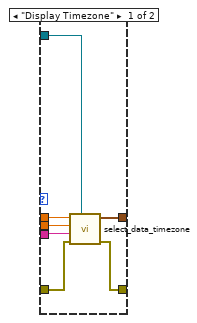
[diagram p9: hidden frame]
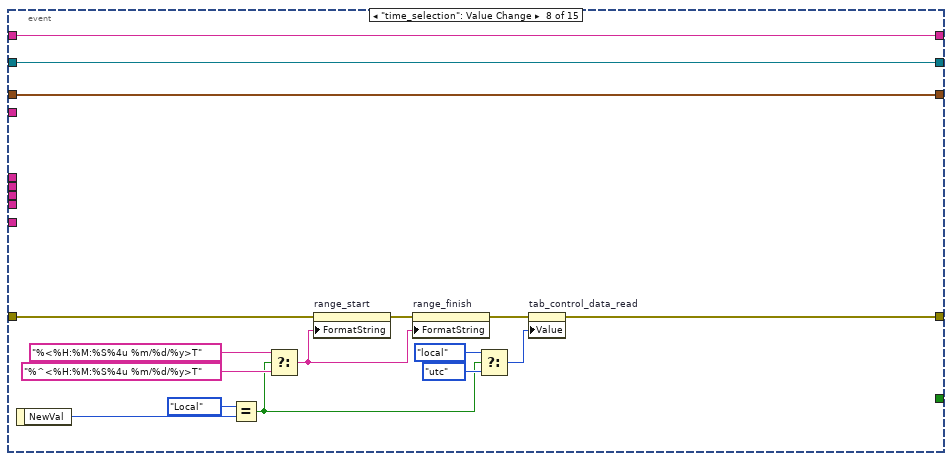
[diagram p10: hidden frame]
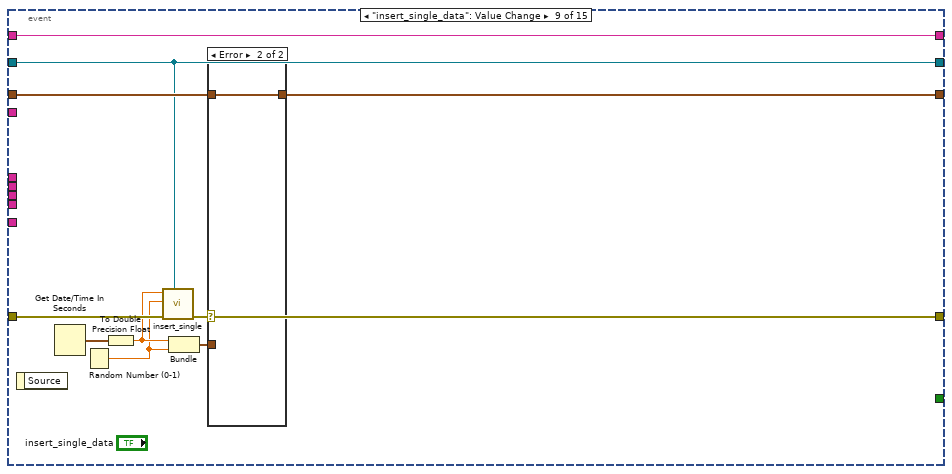
[diagram p11: hidden frame]
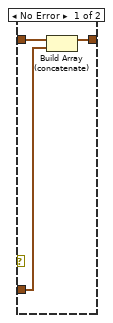
[diagram p12: hidden frame]
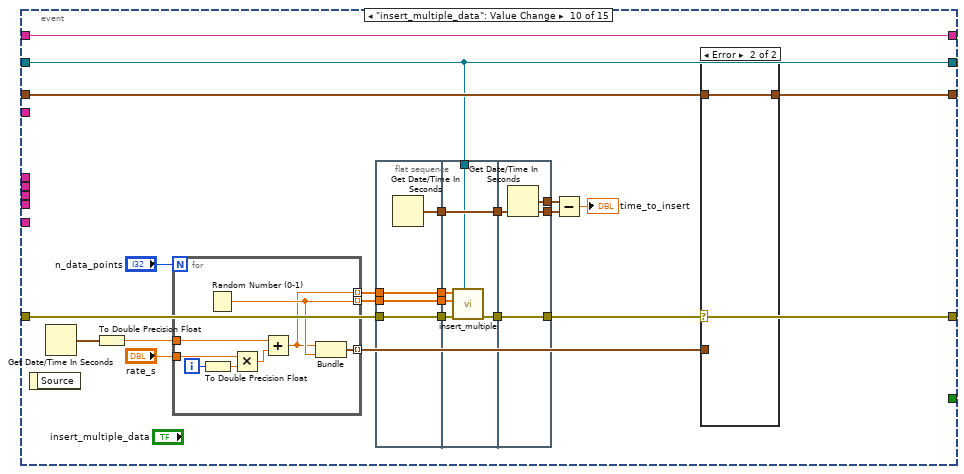
[diagram p13: hidden frame]
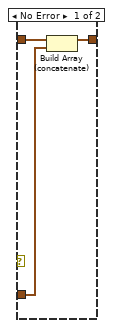
[diagram p14: hidden frame]
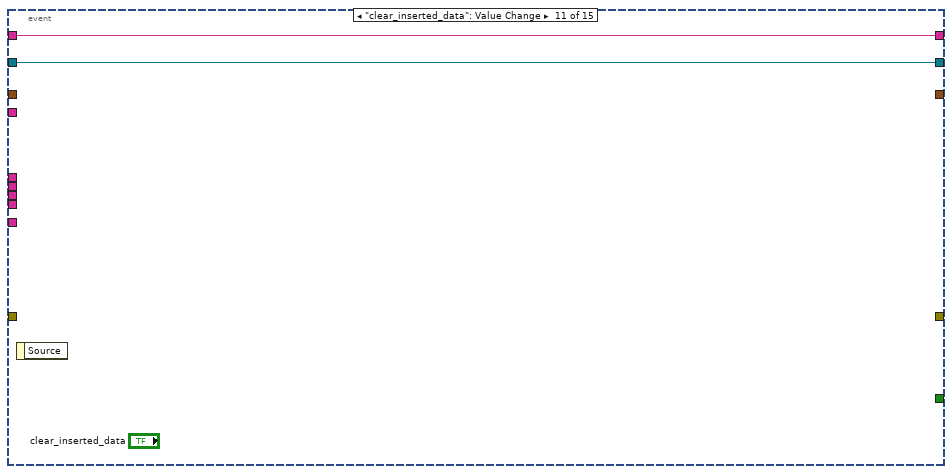
[diagram p15: hidden frame]
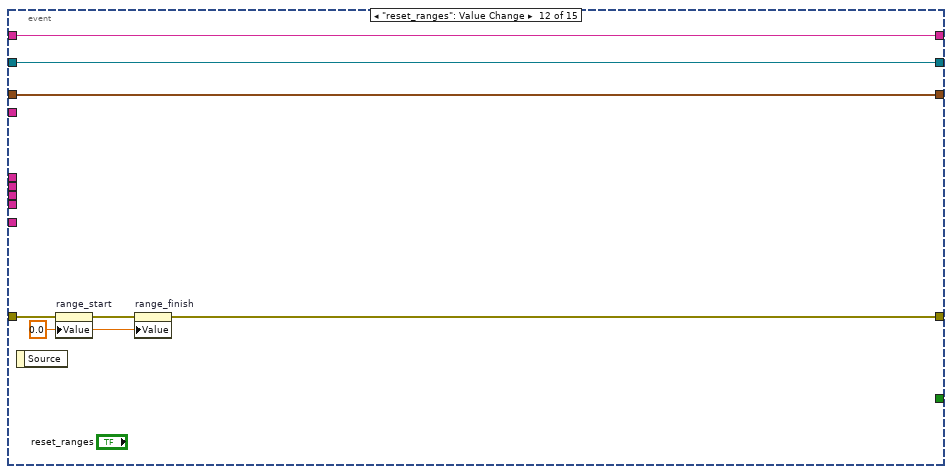
[diagram p16: hidden frame]
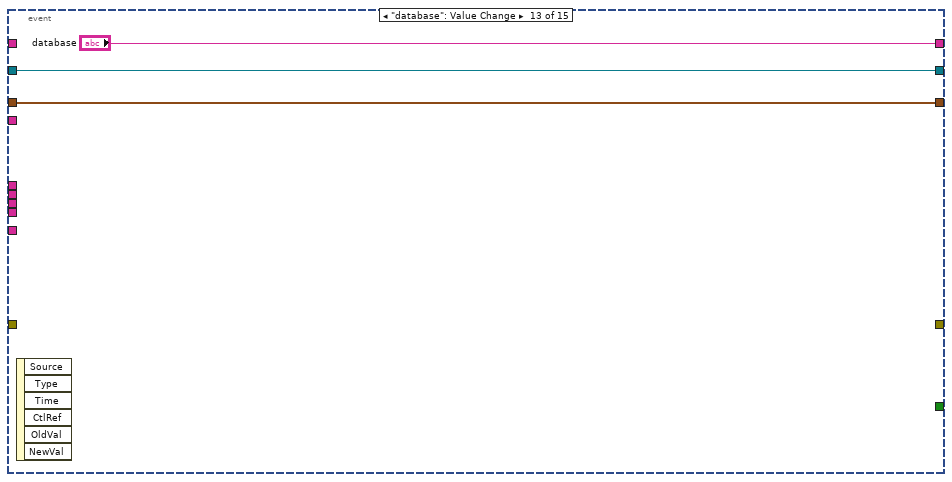
[diagram p17: hidden frame]
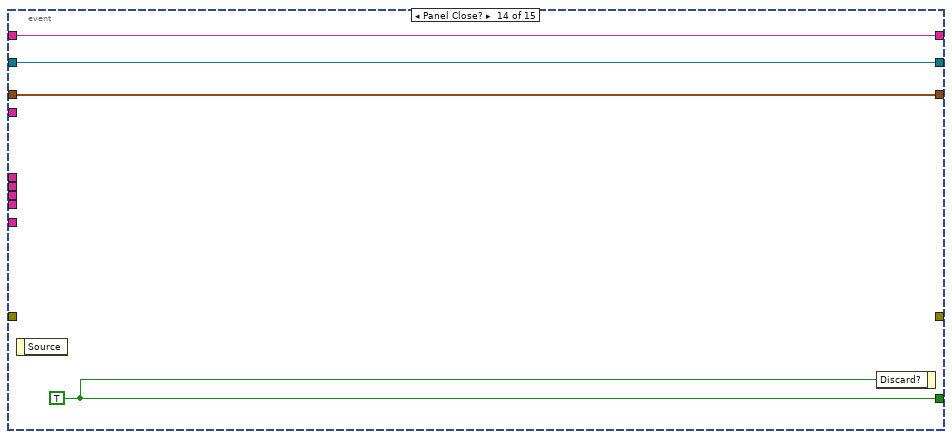
[diagram p18: hidden frame]
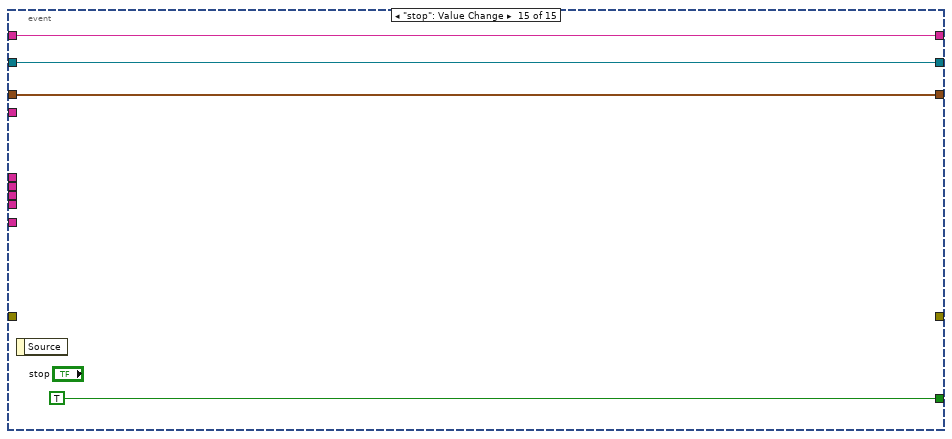
[diagram p19: hidden frame]
diagram:
  w15 = T4 refnum items=["Connection"] ("connection reference")
  n1 = call <vilib>:"Application Directory.vi"() -> ("Application Directory"=w5:path)
  n2 = Build Path(base path=w5, name or relative path=path "sql/lv-example-postgres.sql" ("Application Directory")) -> (appended path=w3:path)
  n3 = Read from Text File(file (use dialog)=w3) -> (text=w2:string)  [unwired: 3 in, 3 out]
  "create_table_sql" <- w2
  n4 = invoke on="connected?" class="Bool (strict)" method="Reinit To Default"() -> (error out=w12:errorcluster)  [unwired: 3 in, 2 out]
  n5 = call "fg_constants.vi"() -> ("table out"=w9:string)  [unwired: 10 in, 1 out]
  n6 = while {
    shift-right: [w27] -> w13
    shift-left: w15 -> [w29]
    tunnel: w12 -> [w26]
    tunnel: w9 -> [w28]
    tunnel: "Driver=%s;Server=%s,%s; Database=%s;" ("connection_string") -> [w25]
    shift-right: [w22] -> _
    shift-left: cluster{"time":dbl, "value":dbl}[] [] ("data_inserted") -> [w24]
    tunnel: "SELECT extract(epoch from now() at time zone 'UTC')" ("table_name") -> [w23]
    tunnel: "SELECT extract(epoch from now() at time zone 'UTC')+2082844800, extract(epoch from now() at time zone ?)+2082844800" ("table_name") -> [w21]
    tunnel: "SHOW timezone;" ("table_name") -> [w20]
    tunnel: [w19] -> w6
    tunnel: w2 -> [w18]
    shift-right: [w16] -> _
    shift-left: "postgres" -> [w17]
    stop <- w30 stop-if-true
    n7 = event shown="[2] \"connect\": Value Change" {
      selector: _ -> [_ _ _ _ _ _ _ _ _ _ _ _ _ _ _]
      dyn-events: _ -> [_ _ _ _ _ _ _ _ _ _ _ _ _ _ _]
      timeout: _ -> [_ _ _ _ _ _ _ _ _ _ _ _ _ _ _]
      tunnel: [_ _ _ _ _ _ _ _ _ _ _ _ _ w281 TRUE] -> w30
      tunnel: [w32 w46 w54 w65 w74 w105 w155 w194 w214 w240 _ w271 _ _ _] -> w19
      tunnel: w29 -> [w33 w41 _ w68 w75 w110 w150 w204 w208 w221 w267 w274 w277 w280 w284]
      tunnel: w28 -> [_ w44 _ _ _ _ _ _ _ _ _ _ _ _ _]
      tunnel: [w33 w41 w59 _ w75 w110 w150 w204 w208 w221 w267 w274 w277 w280 w284] -> w27
      tunnel: w26 -> [w35 w45 w63 w70 w77 w112 w154 w197 w213 w239 _ w273 _ _ _]
      tunnel: w25 -> [_ _ w56 _ _ _ _ _ _ _ _ _ _ _ _]
      tunnel: w24 -> [w36 w40 w55 w69 w101 w121 w149 w203 w211 w237 _ w269 w276 w279 w283]
      tunnel: [w36 w40 w55 w69 w101 w121 w149 w203 w210 w220 _ w269 w276 w279 w283] -> w22
      tunnel: w23 -> [_ _ _ _ _ _ _ _ _ _ _ _ _ _ _]
      tunnel: w21 -> [_ _ _ _ w76 _ _ _ _ _ _ _ _ _ _]
      tunnel: w20 -> [_ _ _ _ _ w111 _ _ _ _ _ _ _ _ _]
      tunnel: w18 -> [w34 _ _ _ _ _ _ _ _ _ _ _ _ _ _]
      tunnel: w17 -> [w31 w39 w50 w64 w71 w102 w130 w189 w205 w219 w266 w268 _ w278 w282]
      tunnel: [w31 w39 w50 w64 w71 w102 w130 w189 w205 w219 w266 w268 "database" w278 w282] -> w16
      event "create_table": Value Change {
        n8 = event-data() -> ()  [unwired: 1 in, 1 out]
        n9 = call-poly <vilib>:"DB Tools Execute Query.vi"("error in (no error)"=w35, "SQL query"=w34, "connection reference"=w33) -> ("error out"=w37:errorcluster, "recordset reference"=w38:T5)  [unwired: 5 in]
        n10 = call-poly <vilib>:"DB Tools Free Object.vi"("error in (no error)"=w37, "recordset reference"=w38) -> ("error out"=w32:errorcluster)  [unwired: 8 in, 1 out]
      }
      event "clear_table": Value Change {
        n11 = event-data() -> ()  [unwired: 1 in, 1 out]
        n12 = Format Into String(format string="DELETE FROM %s", w44) -> (resulting string=w43:string)  [unwired: 2 in, 1 out]
        n13 = call-poly <vilib>:"DB Tools Execute Query.vi"("error in (no error)"=w45, "SQL query"=w43, "connection reference"=w41) -> ("error out"=w47:errorcluster, "recordset reference"=w48:T5)  [unwired: 5 in]
        n14 = call-poly <vilib>:"DB Tools Free Object.vi"("error in (no error)"=w47, "recordset reference"=w48) -> ("error out"=w46:errorcluster)  [unwired: 8 in, 1 out]
      }
      event "connect": Value Change {
        w51 = TRUE ("Value (Signaling)")
        n15 = event-data() -> ()  [unwired: 1 in, 1 out]
        n16 = Format Into String(format string=w56, "driver", "server", "port", w50) -> (resulting string=w62:string)  [unwired: 2 in, 1 out]
        n17 = call-poly <vilib>:"DB Tools Open Connection.vi"("password"="password", "userID"="username", "error in (no error)"=w63, "connection information"=w62) -> ("error out"=w53:errorcluster, "connection reference"=w59:T4)  [unwired: 4 in]
        n18 = property on="connected?" class="Bool (strict)"(error in=w53, "Value"=w51) -> (error out=w52:errorcluster)  [unwired: 1 in, 1 out]
        n19 = property on="get_timezones" class="Bool (strict)"(error in=w52, "Val(Sgnl)"=w51) -> (error out=w54:errorcluster)  [unwired: 1 in, 1 out]
      }
      event "disconnect": Value Change {
        n20 = event-data() -> ()  [unwired: 1 in, 1 out]
        n21 = call <vilib>:"DB Tools Close Connection.vi"("error in (no error)"=w70, "connection reference"=w68) -> ("error out"=w66:errorcluster)  [unwired: 5 in]
        n22 = property on="connected?" class="Bool (strict)"(error in=w66, "Value"=FALSE ("connected?")) -> (error out=w65:errorcluster)  [unwired: 1 in, 1 out]
      }
      event "select_time_now": Value Change {
        n23 = event-data() -> ()  [unwired: 1 in, 6 out]
        n24 = local read "display_timezone"() -> (w85:i32)
        n25 = local read "timezones"() -> (w98:T2[])
        n26 = Index Array(array=w98, index=w85) -> (element=w97:T2)
        n27 = Unbundle By Name(w97) -> ("name"=w78:string)
        n28 = To Variant(anything=w78) -> (Variant=w84:variant)
        n29 = call <vilib>:"DB Tools Parser.vi"("error in (no error)"=w77, "variant"=w84) -> ("error out"=w93:errorcluster, "parameters"=w96:T6[])  [unwired: 2 in]
        n30 = call <vilib>:"DB Tools Create Parameterized Query.vi"("error in (no error)"=w93, "parameters"=w96, "SQL query"=w76, "connection reference"=w75) -> ("error out"=w95:errorcluster, "command reference"=w94:T9)  [unwired: 3 in, 1 out]
        n31 = call-poly <vilib>:"DB Tools Execute Query.vi"("error in (no error)"=w95, "command reference"=w94) -> ("error out"=w89:errorcluster, "command-recordset reference"=w90:T10)  [unwired: 6 in]
        n32 = call-poly <vilib>:"DB Tools Fetch Recordset Data.vi"("error in (no error)"=w89, "command-recordset reference"=w90) -> ("error out"=w100:errorcluster, "recordset data"=w88:variant[][], "command-recordset reference out"=w87:T10)  [unwired: 3 in]
        n33 = Index Array(array=w88, index (row)=0 ("disabled index (col)")) -> (element=w81:variant[])  [unwired: 1 in]
        n34 = call-poly <vilib>:"DB Tools Free Object.vi"("command-recordset reference"=w87) -> ("error out"=w91:errorcluster, "command reference"=w86:T9)  [unwired: 9 in]
        n35 = Variant To Data(error in=w100, type=dbl[] [], Variant=w81) -> (data=w80:dbl[], error out=w99:errorcluster)
        n36 = call-poly <vilib>:"DB Tools Free Object.vi"("command reference"=w86) -> ("error out"=w92:errorcluster)  [unwired: 9 in, 1 out]
        n37 = Merge Errors(w99, w92, w91) -> (w74:errorcluster)
        n38 = To Time Stamp(1:w80) -> (0:w79:timestamp[])
        n39 = Index Array(array=w79) -> (element #1=→"time_local" →"time_utc":timestamp, element #2=→"time_display":timestamp)  [unwired: 2 in]
      }
      event "get_timezones": Value Change {
        w120 = 0 ("index (row)")
        n40 = event-data() -> ()  [unwired: 1 in, 1 out]
        n41 = call-poly <vilib>:"DB Tools Execute Query.vi"("error in (no error)"=w112, "SQL query"=w111, "connection reference"=w110) -> ("error out"=w116:errorcluster, "recordset reference"=w117:T5)  [unwired: 5 in]
        n42 = call-poly <vilib>:"DB Tools Fetch Recordset Data.vi"("error in (no error)"=w116, "recordset reference"=w117) -> ("error out"=w124:errorcluster, "recordset data"=w114:variant[][], "recordset reference out"=w118:T5)  [unwired: 3 in]
        n43 = Index Array(array=w114, index (row)=w120, index (col)=w120) -> (element=w119:variant)
        n44 = invoke on="get_timezones" class="Bool (strict)" method="Reinit To Default"() -> ()  [unwired: 3 in, 3 out]
        n45 = Variant To Data(error in=w124, type="" ("Array"), Variant=w119) -> (data=→"server_timezone":string, error out=w123:errorcluster)
        n46 = call-poly <vilib>:"DB Tools Free Object.vi"("error in (no error)"=w123, "recordset reference"=w118) -> ("error out"=w103:errorcluster)  [unwired: 8 in, 1 out]
        n47 = call "select_timezones.vi"("connection_reference"=w110, "error in (no error)"=w103) -> ("error out"=w122:errorcluster, "timezones"=w109:T2[])  [unwired: 8 in]
        "timezones" <- w109
        n48 = for {
          tunnel: w109 -> [w129] mode=indexing
          tunnel: [w128] -> w106 mode=indexing
          n49 = Unbundle By Name(w129) -> ("name"=w127:string, "utc_offset"=w126:dbl)
          n50 = Format Into String(format string="%s (%<%H:%M:%S>t)", w127, w126) -> (resulting string=w128:string)  [unwired: 2 in, 1 out]
        }
        n51 = property on="display_timezone" class="Ring (strict)"(error in=w122, "Strings []"=w106) -> (error out=w104:errorcluster)  [unwired: 1 in, 1 out]
        n52 = call "find_timezones.vi"("error in (no error)"=w104, "timezones []"=w109) -> ("error out"=w105:errorcluster, "timezone_offset"=→"timezone_offset":dbl, "timezone_names []"=→"timezone_names []":string[])  [unwired: 7 in]
      }
      event "read_data": Value Change {
        n53 = event-data() -> ()  [unwired: 1 in, 1 out]
        n54 = local read "timezones"() -> (w147:T2[])
        n55 = Index Array(array=w147, index="display_timezone") -> (element=w146:T2)
        n56 = Unbundle By Name(w146) -> ("name"=w144:string)
        n57 = flat-sequence {
          tunnel: w144 -> [w157]
          tunnel: "time_selection" -> [w158]
          tunnel: w150 -> [w159]
          tunnel: "range_finish" -> [w160]
          tunnel: "range_start" -> [w161]
          tunnel: w154 -> [w162]
          tunnel: [w162] -> w141
          tunnel: [w161] -> w140
          tunnel: [w160] -> w139
          tunnel: [w159] -> w138
          tunnel: [w158] -> w137
          tunnel: [w157] -> w136
          tunnel: [w156] -> w135
          tunnel: [w171] -> w143
          tunnel: [w166] -> w142
          tunnel: w141 -> [w170]
          tunnel: w140 -> [w169]
          tunnel: w139 -> [w168]
          tunnel: w138 -> [w167]
          tunnel: w137 -> [w165]
          tunnel: w136 -> [w164]
          tunnel: w135 -> [w163]
          tunnel: [w163] -> w134
          tunnel: [w187] -> w148
          tunnel: [w188] -> w155
          tunnel: w143 -> [w188]
          tunnel: w142 -> [w187]
          tunnel: [w186] -> w133
          tunnel: w134 -> [w185]
          tunnel: [w185] -> w132
          frame #0 {
            n58 = Get Date/Time In Seconds() -> (seconds since 1Jan1904=w156:timestamp)
          }
          frame #1 {
            n59 = case shown="Default" w165 {
              tunnel: [w174 w184] -> w171
              tunnel: w170 -> [w173 w183]
              tunnel: w169 -> [w178 w182]
              tunnel: w168 -> [w177 w181]
              tunnel: w167 -> [w176 w180]
              tunnel: [w175 w179] -> w166
              tunnel: w164 -> [w172 _]
              frame "Display Timezone" {
                n60 = call "select_data_timezone.vi"("connection_reference"=w176, "error in (no error)"=w173, "timezone"=w172, "range_finish"=w177, "range_start"=w178) -> ("error out"=w174:errorcluster, "data_read"=w175:cluster{"time":dbl, "value":dbl}[])  [unwired: 5 in]
              }
              frame Default {
                n61 = call "select_data.vi"("connection_reference"=w180, "error in (no error)"=w183, "range_finish_utc"=w181, "range_start_utc"=w182) -> ("error out"=w184:errorcluster, "data_read"=w179:cluster{"time":dbl, "value":dbl}[])  [unwired: 6 in]
              }
            }
          }
          frame #2 {
            n62 = Get Date/Time In Seconds() -> (seconds since 1Jan1904=w186:timestamp)
          }
        }
        n63 = Subtract(x=w133, y=w132) -> (x-y=→"time_to_read":dbl)
        "data_read_utc" <- w148
        "data_read_local" <- w148
      }
      event "time_selection": Value Change {
        n64 = event-data() -> ("NewVal"=w202:T3)  [unwired: 1 in]
        n65 = Equal?(x=T3."Local" ("y"), y=w202) -> (x = y?=w190:bool)
        n66 = Select(t="%<%H:%M:%S%4u %m/%d/%y>T", s=w190, f="%^<%H:%M:%S%4u %m/%d/%y>T") -> (s? t:f=w198:string)
        n67 = property on="range_start" class="DigNum (strict)"(error in=w197, "FormatString"=w198) -> (error out=w196:errorcluster)  [unwired: 1 in, 1 out]
        n68 = property on="range_finish" class="DigNum (strict)"(error in=w196, "FormatString"=w198) -> (error out=w195:errorcluster)  [unwired: 1 in, 1 out]
        n69 = Select(t=enum32{"utc", "local"}."local" ("tab_control_data_read"), s=w190, f=enum32{"utc", "local"}."utc" ("tab_control_data_read")) -> (s? t:f=w192:enum32{"utc", "local"})
        n70 = property on="tab_control_data_read" class="TabCtl (strict)"(error in=w195, "Value"=w192) -> (error out=w194:errorcluster)  [unwired: 1 in, 1 out]
      }
      event "insert_single_data": Value Change {
        n71 = event-data() -> ()  [unwired: 1 in, 1 out]
        n72 = Get Date/Time In Seconds() -> (seconds since 1Jan1904=w212:timestamp)
        n73 = Random Number (0-1)() -> (number: 0 to 1=w206:dbl)
        n74 = To Double Precision Float(number=w212) -> (double precision float=w207:dbl)
        n75 = call "insert_single.vi"("connection_reference"=w208, "error in (no error)"=w213, "value"=w206, "date_time"=w207) -> ("error out"=w214:errorcluster)  [unwired: 7 in]
        n76 = Bundle(w207, "number: 0 to 1"=w206) -> (w209:cluster{dbl, "number: 0 to 1":dbl})  [unwired: 1 in]
        n77 = case shown="Error" w214 {
          tunnel: w211 -> [w217 w218]
          tunnel: [w216 w218] -> w210
          tunnel: w209 -> [w215 _]
          frame No Error {
            n78 = Build Array (concatenate)(w217, w215) -> (w216:cluster{"time":dbl, "number: 0 to 1":dbl}[])
          }
          frame Error {
          }
        }
      }
      event "insert_multiple_data": Value Change {
        n79 = event-data() -> ()  [unwired: 1 in, 1 out]
        n80 = Get Date/Time In Seconds() -> (seconds since 1Jan1904=w238:timestamp)
        n81 = To Double Precision Float(number=w238) -> (double precision float=w233:dbl)
        n82 = for {
          N: "n_data_points" -> [_]
          tunnel: [w261] -> w236 mode=indexing
          tunnel: [w260] -> w235 mode=indexing
          tunnel: w233 -> [w258]
          tunnel: "rate_s" -> [w256]
          tunnel: [w255] -> w231 mode=indexing
          i -> [w257]
          n83 = To Double Precision Float(number=w257) -> (double precision float=w254:dbl)
          n84 = Random Number (0-1)() -> (number: 0 to 1=w261:dbl)
          n85 = Multiply(x=w256, y=w254) -> (x*y=w259:dbl)
          n86 = Add(x=w258, y=w259) -> (x+y=w255:dbl)
          n87 = Bundle(w255, "number: 0 to 1"=w261) -> (w260:cluster{dbl, "number: 0 to 1":dbl})  [unwired: 1 in]
        }
        n88 = flat-sequence {
          tunnel: w231 -> [w242]
          tunnel: w236 -> [w243]
          tunnel: w239 -> [w244]
          tunnel: [w244] -> w229
          tunnel: [w243] -> w228
          tunnel: [w242] -> w227
          tunnel: [w241] -> w226
          tunnel: [w250] -> w230
          tunnel: w229 -> [w249]
          tunnel: w228 -> [w245]
          tunnel: w227 -> [w246]
          tunnel: w226 -> [w248]
          tunnel: [w248] -> w225
          tunnel: w221 -> [w247]
          tunnel: [w253] -> w240
          tunnel: w230 -> [w253]
          tunnel: [w252] -> w224
          tunnel: w225 -> [w251]
          tunnel: [w251] -> w223
          frame #0 {
            n89 = Get Date/Time In Seconds() -> (seconds since 1Jan1904=w241:timestamp)
          }
          frame #1 {
            n90 = call "insert_multiple.vi"("connection_reference"=w247, "error in (no error)"=w249, "value []"=w245, "date_time []"=w246) -> ("error out"=w250:errorcluster)  [unwired: 7 in]
          }
          frame #2 {
            n91 = Get Date/Time In Seconds() -> (seconds since 1Jan1904=w252:timestamp)
          }
        }
        n92 = Subtract(x=w224, y=w223) -> (x-y=→"time_to_insert":dbl)
        n93 = case shown="Error" w240 {
          tunnel: w237 -> [w264 w265]
          tunnel: [w263 w265] -> w220
          tunnel: w235 -> [w262 _]
          frame No Error {
            n94 = Build Array (concatenate)(w264, w262) -> (w263:cluster{"time":dbl, "number: 0 to 1":dbl}[])
          }
          frame Error {
          }
        }
      }
      event "clear_inserted_data": Value Change {
        n95 = event-data() -> ()  [unwired: 1 in, 1 out]
      }
      event "reset_ranges": Value Change {
        w270 = 0.0 ("range_start")
        n96 = event-data() -> ()  [unwired: 1 in, 1 out]
        n97 = property on="range_start" class="DigNum (strict)"(error in=w273, "Value"=w270) -> (error out=w272:errorcluster)  [unwired: 1 in, 1 out]
        n98 = property on="range_finish" class="DigNum (strict)"(error in=w272, "Value"=w270) -> (error out=w271:errorcluster)  [unwired: 1 in, 1 out]
      }
      event "database": Value Change {
        n99 = event-data() -> ()  [unwired: 1 in, 6 out]
      }
      event Panel Close? {
        w281 = TRUE
        n100 = event-data() -> ()  [unwired: 1 in, 1 out]
        n101 = event-data("Discard?"=w281) -> ()  [unwired: 1 in, 1 out]
      }
      event "stop": Value Change {
        n102 = event-data() -> ()  [unwired: 1 in, 1 out]
      }
    }
    "data_inserted" <- w22
    n103 = local write "error"(w19) -> ()
  }
  n104 = call <vilib>:"DB Tools Close Connection.vi"("connection reference"=w13) -> ()  [unwired: 6 in, 1 out]
  n105 = disable-structure shown="RUN_TIME_ENGINE==True" {
    disable-tunnel: w6 -> [_ w287]
    frame condition #0 {
      n106 = Quit LabVIEW(quit? (T)=TRUE) -> ()
    }
    frame condition #1 (active) {
      "error" <- w287
    }
  }
